vi "controllerFPGA_multiTarget.vi"() -> ()   [LabVIEW 2016]
uses:
  <vilib>/Platform/TimedLoop/XDataNode/timing_clust.ctl
  <vilib>/Platform/TimedLoop/XDataNode/nitl_modes.ctl
  <vilib>/Platform/TimedLoop/XDataNode/wakeup.ctl
  <vilib>/rvi/Emulation/niFpgaGetClockAttributes.vi
  <vilib>/rvi/Emulation/niFpgaSctlEmulationGetInTimedLoop.vi
  <vilib>/rvi/Emulation/niFpgaEmulationReportErrorSimple.vi
  <vilib>/rvi/Memory/Memory_Emulation/nirvimemoryFastEmulation.vi
  <vilib>/rvi/Memory/Memory_Emulation/nirvimemoryEmulation.vi
  <vilib>/rvi/Emulation/niFpgaEmulationIsFPGAContextNoSignature.vi
  <vilib>/rvi/DataTransferAndStorage/Container/Common/niFpgaContainerGetUniqueNameForEmu.vi
  <vilib>/rvi/Emulation/niFpgaProcessEmulError.vi
  <vilib>/rvi/errors/nirviReportUnexpectedCaseInternalError (U32).vi
  <vilib>/rvi/Emulation/niFpgaCriticalErrorInLSC.vi
  <vilib>/rvi/errors/niFpgaSetErrorForExecOnDevCompSimple.vi
  <vilib>/rvi/eio/common/nirviEmuReportErrorAndStop.vi
  <vilib>/rvi/FIFO/Fifo_Resource/nirvififoEmulationSetSize.vi
  <vilib>/rvi/FIFO/Fifo_Resource/nirviFifoEmulationQueueMgr.vi
  <instcachedir>/0/nirviFifoEmulationQueueMgr_E5CAEC123FF24DC58D834DCA3CDAA9B5.lvgen/nirviFifoEmulationQueueMgr_E5CAEC123FF24DC58D834DCA3CDAA9B5_010.vi
  <vilib>/Utility/error.llb/Clear Errors.vi
  <vilib>/rvi/FIFO/Fifo_Resource/nirvififoEmulationCreateLock.vi
  <vilib>/rvi/FIFO/Fifo_Resource/nirvififoEmulationObtainLock.vi
  <vilib>/rvi/FIFO/Fifo_Resource/nirvififoEmulationReleaseLock.vi
  <vilib>/rvi/occurrence/nirviWaitOnOccurrenceBase.vi
  <vilib>/rvi/errors/nirviReportUnexpectedCaseInternalError.vi
  <vilib>/rvi/FIFO/Fifo_Resource/nirvififoEmulationDetermineInputValidOut.vi
  <vilib>/rvi/Memory/Memory_Emulation/niFpgaMemoryEmulationCacheClearOnFirstRun.vi
  <vilib>/rvi/Memory/Memory_Emulation/nirvimemoryEmulationManagerCache_MakeExclusive.vi
  <vilib>/rvi/Memory/Memory_Emulation/niFpgaMemoryEmulationValidateCache.vi
  <vilib>/rvi/Memory/Memory_Emulation/nirvimemoryEmulationManagerCache_InsertValue.vi
  <vilib>/rvi/Memory/Memory_Emulation/nirvimemoryEmulationManagerCache_ReleaseExclusive.vi
  <vilib>/rvi/Memory/Memory_Emulation/nirvimemoryEmulationManagerCache_GetValue.vi
  <vilib>/rvi/Memory/Memory_Emulation/nirvimemoryEmulationManagerCache_SetValue.vi
  <vilib>/rvi/eio/common/nirviEmuTemplateMethod_errors.vi
  <instcachedir>/0/nirviFifoEmulationQueueMgr_E5CAEC123FF24DC58D834DCA3CDAA9B5.lvgen/nirviFifoEmulationQueueMgr_E5CAEC123FF24DC58D834DCA3CDAA9B5_009.vi
  <instcachedir>/0/nirviFifoEmulationQueueMgr_E5CAEC123FF24DC58D834DCA3CDAA9B5.lvgen/nirviFifoEmulationQueueMgr_E5CAEC123FF24DC58D834DCA3CDAA9B5_021.vi
  <instcachedir>/0/nirviFifoEmulationQueueMgr_E5CAEC123FF24DC58D834DCA3CDAA9B5.lvgen/nirviFifoEmulationQueueMgr_E5CAEC123FF24DC58D834DCA3CDAA9B5_014.vi
  <vilib>/rvi/interface/RandomDataEmulation/niFpgaRandomDataHandleErrors.vi
  <instcachedir>/0/nirviFifoEmulationQueueMgr_E5CAEC123FF24DC58D834DCA3CDAA9B5.lvgen/nirviFifoEmulationQueueMgr_E5CAEC123FF24DC58D834DCA3CDAA9B5_036.vi
  <instcachedir>/0/nirviFifoEmulationQueueMgr_E5CAEC123FF24DC58D834DCA3CDAA9B5.lvgen/nirviFifoEmulationQueueMgr_E5CAEC123FF24DC58D834DCA3CDAA9B5_035.vi
  <vilib>/rvi/eio/common/nirviEmuTemplatePropertySet_noerrors.vi
  <instcachedir>/0/nirviFifoEmulationQueueMgr_E5CAEC123FF24DC58D834DCA3CDAA9B5.lvgen/nirviFifoEmulationQueueMgr_E5CAEC123FF24DC58D834DCA3CDAA9B5_003.vi
  <instcachedir>/0/nirviFifoEmulationQueueMgr_E5CAEC123FF24DC58D834DCA3CDAA9B5.lvgen/nirviFifoEmulationQueueMgr_E5CAEC123FF24DC58D834DCA3CDAA9B5_000.vi
  <instcachedir>/0/nirviFifoEmulationQueueMgr_E5CAEC123FF24DC58D834DCA3CDAA9B5.lvgen/nirviFifoEmulationQueueMgr_E5CAEC123FF24DC58D834DCA3CDAA9B5_032.vi
  <instcachedir>/0/nirviFifoEmulationQueueMgr_E5CAEC123FF24DC58D834DCA3CDAA9B5.lvgen/nirviFifoEmulationQueueMgr_E5CAEC123FF24DC58D834DCA3CDAA9B5_007.vi
  <instcachedir>/0/nirviFifoEmulationQueueMgr_E5CAEC123FF24DC58D834DCA3CDAA9B5.lvgen/nirviFifoEmulationQueueMgr_E5CAEC123FF24DC58D834DCA3CDAA9B5_011.vi
  <instcachedir>/0/nirviFifoEmulationQueueMgr_E5CAEC123FF24DC58D834DCA3CDAA9B5.lvgen/nirviFifoEmulationQueueMgr_E5CAEC123FF24DC58D834DCA3CDAA9B5_004.vi
  <instcachedir>/0/nirviFifoEmulationQueueMgr_E5CAEC123FF24DC58D834DCA3CDAA9B5.lvgen/nirviFifoEmulationQueueMgr_E5CAEC123FF24DC58D834DCA3CDAA9B5_033.vi
  <vilib>/rvi/DataTransferAndStorage/Container/XNode/niFpgaContainer.xnode
  <vilib>/Platform/TimedLoop/XDataNode/XDataNode.xnode
  <vilib>/rvi/FIFO/Fifo_Resource/nirvififoEmulationRead.vi
  <vilib>/rvi/FXPMathLib/FxpInterpret/XNode/nifxpmath_Interpret.xnode
  <vilib>/rvi/FIFO/Fifo_Resource/nirvififoEmulationWrite.vi
  <vilib>/rvi/DataTransferAndStorage/Register/Emulation/niFpgaRegisterEmulation.vi
  <vilib>/eio/EIONode/EIONode.xnode
  <vilib>/rvi/interface/RandomDataEmulation/nirviRandomDataFpgaReadWriteTemplate.vi
  <vilib>/eio/EIOPropertyNode/EIOPropertyNode.xnode
  <vilib>/rvi/DataTransferAndStorage/Handshake/Emulation/niFpgaHandshakeEmulation.vi
  <vilib>/rvi/FXPMathLib/FxpAdd/XNode/nifxpmath_Add.xnode
  <vilib>/Platform/TimedLoop/XDataNode/XDNodeRunTimeDep.lvlib
  <instrlib>/_niInstr/Basic Elements/v1/FPGA/niInstr Basic Elements v1 FPGA.lvlib
  <vilib>/rvi/FXPMathLib/sim/FxpSim.dll
  <vilib>/rvi/eio/common/nirviEmuTemplatePropertyGet_errors.vi
  <vilib>/rvi/eio/common/nirviEmuTemplatePropertyGet_noerrors.vi
  <vilib>/rvi/eio/common/nirviEmuTemplatePropertySet_errors.vi
  <vilib>/rvi/Memory/Memory_Emulation/niFpgaMemoryEmulationDramRetrieveData.vi
  <vilib>/rvi/Memory/Memory_Emulation/niFpgaMemoryFastEmulationDramWriteAndRequestData.vi
  <vilib>/rvi/Memory/Memory_Emulation/niFpgaMemoryEmulationDramWriteAndRequestData.vi
panel:
  in  "dio.i.dataIn":bool
  in  "dio.p.multiplexerOE":bool
  in  "dio.p.multiplexerclock":bool
  in  "dio.p.multiplexerSync":bool
  in  "dio.p.multiplexerReset":bool
  in  "se.tabs":T1(tab)
  in  "se.p.closedLoop":bool
  in  "se.p.scanSize":T2
  in  "se.p.transformMatrix":T3
  in  "se.p.scanOffsets":cluster{"x":fxp<+/-,16,1>, "y":fxp<+/-,16,1>}
  in  "se.p.clocks":T4={"outputRate"=50, "fastDecFactor"=0, "outWaveSizeFast"=0, "pplUpsampling"=0, "numLines"=0, "se.p.fastInvDec"=0.0, "se.p.slowUpStep"=0.0, "se.p.outWaveSizeSlow"=0, "blankingMax"=10000000, "se.p.fastBlanking"={"startFwd"=0, "endFwd"=10000, "startBwd"=0, "endBwd"=0, "disableBlanking"=FALSE, "useCoarseCounter"=TRUE}}
  in  "se.p.modes":T5
  in  "se.m.slowAxis":T6
  in  "se.m.fastAxis":T6
  out "se.s.realXYOutputRate":u32
  out "se.s.blankingOff":bool
  out "se.o.position":T7
  out "clocksOut":T8
  in  "se.p.durationTrigger":u16=100
  in  "se.p.y.fbParams":T9={"enable"=FALSE, "setPoint"=0.001007080078125, "pGain"=0.0, "iGain"=0.10000038146972656, "gainScale"=0}
  in  "se.p.x.fbParams":T9={"enable"=FALSE, "setPoint"=0.001007080078125, "pGain"=0.0, "iGain"=0.10000038146972656, "gainScale"=0}
  in  "se.mot.p.target":cluster{"x":fxp<+/-,16,1>, "y":fxp<+/-,16,1>}
  out "se.mot.s.running":bool
  in  "se.mot.p.clocks":T10
  in  "se.mot.m.motion":T11
  out "se.mot.s.origin":T12
  in  "se.sid.prbs":cluster{"write":bool, "index":u16, "data":bool}
  in  "se.sid.start":bool
  in  "se.sid.p.axisXNotY":bool=TRUE
  in  "se.sid.p.params":T13={"sysIdOutputRate"=100, "sysIdWaveSize"=4092, "sysIdRepetitions"=50, "high"=0.0, "low"=0.0} {"sysIdOutputRate" min=10}
  out "se.sid.s.repetitions":u16
  out "se.sid.s.running":bool
  in  "stepmot.delay(ms)":u16
  in  "stepmot.dir":bool
  in  "stepmot.enable":bool
  in  "stepmot.on":bool
  in  "stepmot.steps":u16
  in  "smd.address":i8
  in  "smd.p.writeMem":T14={"write"=FALSE, "index"=0, "data"=[TRUE, FALSE, FALSE, FALSE]}
  out "stepmot.running":bool
  in  "ort.bgc.requestType":i16(ring) items=["Never", "EndOfLine", "EndOfFrame"]
  in  "aio.wfm.enable":bool
  out "aio.s.slowActualOutputRate":u32
  in  "wfm.rampRange":T15
  in  "wfm.Parameters":T16
  in  "wfm.initialPositions":T17
  in  "wfm.reset":cluster{"rampx":bool, "ustepx":bool}
  out "wfm.displacementFinished":bool
  out "wfm.microStepIndex":cluster{"CurrentUstep":i16, "NextUstep":i16}
  out "wfm.rampIndex":cluster{"ramp index":i16, "NextRamp":i16}
  in  "Tab Control":T18(tab)
  in  "aio.o.fastInput":bool
  in  "aio.o.invertHeight":bool
  out "aio.o.inputs":i16[](array[numeric])
  out "aio.s.HSaux":fxp<+/-,24,16>
  in  "aio.i.slowInputRate":u16 caption="Count(Ticks)"
  out "aio.s.slowVertical":i16
  out "aio.s.sum":i16
  out "aio.s.slowHoriz":i16
  in  "aio.o.bypassDither":bool
  in  "aio.m.drive":cluster{"write":bool, "data":i16, "index":u16}
  in  "aio.o.disableExc":bool=TRUE
  out "aio.s.clock":refnum<k21>
  out "aio.s.slowActualInputRate":u32
  out "aio.s.slowActualFBOutRate":u32
  in  "aio.o.invertOutputs":bool[](array[boolean])=[FALSE, FALSE, FALSE, FALSE, FALSE, FALSE, FALSE, FALSE]
  in  "aio.o.outputs":i16[](array[numeric])=[0, 0, 0, 0]
  in  "aio.o.invertInputs":bool[](array[boolean])=[FALSE, FALSE, FALSE, FALSE, FALSE, FALSE, FALSE, FALSE]
  in  "aio.o.invert2Inputs":bool[](array[boolean])=[FALSE, FALSE]
  in  "aio.i.samplingDecimation":u16=1
  in  "AI.voltage Range":T19(ring)
  in  "aio.p.fastADCclockdec":u16
  out "aio.s.fastVertical":i16
  out "aio.s.fastHoriz":i16
  in  "aio.o.heightLimits":cluster{"upper":i16, "lower":i16}={"upper"=32767, "lower"=-32768}
  in  "aio.flt.bypass":bool[](array[boolean])=[TRUE, TRUE, TRUE, TRUE]
  in  "aio.flt.p.anot4x":fxp<+/-,24,8>[](array[numeric])=[0.0, 0.0, 0.0, 0.0, 0.0, 0.0, 0.0, 0.0]
  in  "aio.flt.p.b4x":fxp<+/-,24,8>[](array[numeric])=[0.0, 0.0, 0.0, 0.0, 0.0, 0.0, 0.0, 0.0, 0.0, 0.0, 0.0, 0.0]
  in  "hdt.aux.o.enable":bool
  in  "hdt.o.enable":bool=TRUE
  out "hdt.o.overflow":bool
  out "hdt.o.ticksPerPixel":u32
  in  "hdt.mainOutStreamSelect":u8(ring) items=["PID/ORT", "SICM"]
  out "hdt.int.s.debug":T20
  in  "hdt.int.p.memWriteSource":u8(ring) items=["ORT", "SICM"]
  out "hdt.int.s.dataLost":bool
  in  "hdt.int.s.clearDataLost":bool
  in  "hdt.int.p.readParams":T21={"hdt.int.s.transferSource"=0, "hdt.int.p.useInternalMemStartPos"=FALSE, "hdt.int.p.memStartPos"=0.0, "hdt.int.p.readLength"=100, "hdt.int.p.readFwd"=TRUE, "hdt.int.p.memReadDec"=10, "hdt.int.p.startTransfer"=TRUE} {"hdt.int.s.transferSource" items=["memoryChan1", "memoryChan2", "processVarFixedNoPts", "processVarStream", "systemId", "interleaveMemCh1Ch2"]}
  out "hdt.debugStream":T22
  in  "hdt.p.mainAverageEnabled":bool=TRUE
  in  "fb.p.limits":T23={"upperLimit"=1.0, "lowerLimit"=-1.0}
  in  "fb.i.source":u8(ring) items=["Contact Mode", "ORT", "Aux"]
  in  "fb.p.enable":bool
  in  "fb.p.params":T24={"setPoint"=0.001007080078125, "pGain"=0.0, "iGain"=0.10000038146972656, "gainScale"=3, "setPointAlt"=0.001007080078125}
  in  "fb.loff.p.params":T25={"liftHeight"=0.0498046875, "disengagePos"=-1.0}
  out "fb.s.atLimit":bool
  out "fb.i.rescaled":fxp<+/-,24,1> format="%#_6p"
  out "fb.i.raw":fxp<+/-,24,16>
  in  "fb.p.allowSetpointSwitch":bool
  out "fb.mot.s.running":bool
  out "fb.o.height":fxp<+/-,31,4>
  in  "fb.mot.m.motion":T26
  in  "fb.zWatchdogArm":bool=TRUE
  in  "fb.p.zWatchDogTreshold":fxp<+/-,20,2>
  in  "fb.mot.p.params":T27
  in  "ort.p.waveSize":u16=5000
  in  "ort.o.piezoMode":bool
  in  "ort.p.methodParams":T28={"ort.p.winSizeP2"=2, "ort.p.syncPoint"=0, "ort.p.useSyncPoint"=FALSE, "ort.p.bypassAvg"=FALSE, "ort.p.searchBounds"={"maxSearchLower"=200, "maxSearchUpper"=600}}
  out "ort.o.maxIndex":u16
  in  "ort.p.fcAvgEnable":bool
  in  "ort.p.fcAvg":i8=-4
  in  "ort.bgc.p.scannerTc":u32=1000 caption="scanner Time Constant [us]"
  in  "ort.bgc.p.start":bool
  in  "ort.bgc.p.bgCntP2":u16=12
  in  "ort.bgc.p.waitTicks":u32
  in  "itc.p.allowBGC":bool
  out "aio.s.ortSubstDeflection":cluster{"index":u16, "data":i16}
  out "ort.o.interactionMax":fxp<+/-,24,16>
  in  "ort.fit.p.params":T29={"maxLoc"=0, "threshold"=0, "fitHardPtLimit"=5000}
  in  "ort.fit.m.coefficients":T30
  in  "ort.fit.m.weights":T31
  in  "hsdc.p.points":u32
  in  "hsdc.p.start":bool
  in  "hsdc.o.address":u32
  out "hsdc.o.read":T32
  in  "hsdc.p.substBgnd":bool=TRUE
  in  "sid.m.motion":cluster{"write":bool, "data":bool, "index":u16}
  out "sid.s.running":bool
  out "sid.o.count":u16
  in  "sid.p.start":bool
  in  "sid.p.params":T33={"sysIdOutputRate"=100, "sysIdWaveSize"=4092, "sysIdRepetitions"=50, "lowValue"=0.0, "highValue"=0.010009765625} {"sysIdOutputRate" min=10}
  in  "sid.allowExternalRecord":bool=TRUE
  in  "sid.p.idSource":u8(ring) items=["error", "height"]
  in  "sicm.m.upMotion":T26
  out "sicm.o.height":fxp<+/-,28,2>
  in  "sicm.blc.p.params":T34={"se.blc.p.postRetractDelay"=0, "se.blc.p.windowSize"=0, "se.blc.p.updateFactor"=-8, "blc.resetBackground"=FALSE, "se.blc.p.mindelta"=3.0502676963806152e-05}
  in  "sicm.p.clocks":T35
  in  "sicm.p.params":T36={"sicm.p.setPoint"=0.9999847412109375, "sicm.p.setPointFrac"=1.0, "stepDown"=0.0, "retractHeight"=0.0, "adaptiveMin"=0.0} {"sicm.p.setPoint" format="%#_3g"}
  in  "sicm.display":T37
  in  "sicm.p.modes":T38
  out "sicm.Debug":T39
  out "sicm.s.baseline":T40
  out "sicm-hdt.t.triggerHeight":fxp<+/-,22,4>
  out "flt.o.height":fxp<+/-,20,2>
  in  "flt.ss.p.enable":bool
  in  "flt.ss.p.rate":u16=1000
  in  "flt.bypass1":bool[](array[boolean])=[TRUE, TRUE, TRUE, TRUE, TRUE, TRUE, TRUE, TRUE]
  in  "flt.bypass2":bool[](array[boolean])=[TRUE, TRUE, TRUE, TRUE]
  in  "flt.p.anot8x":fxp<+/-,24,8>[](array[numeric])=[0.0, 0.0, 0.0, 0.0, 0.0, 0.0, 0.0, 0.0, 0.0, 0.0, 0.0, 0.0, 0.0, 0.0, 0.0, 0.0]
  in  "flt.p.b8x":fxp<+/-,24,8>[](array[numeric])=[0.0, 0.0, 0.0, 0.0, 0.0, 0.0, 0.0, 0.0, 0.0, 0.0, 0.0, 0.0, 0.0, 0.0, 0.0, 0.0, 0.0, 0.0, 0.0, 0.0, 0.0, 0.0, 0.0, 0.0]
  in  "flt.p.anot4x":fxp<+/-,24,8>[](array[numeric])=[0.0, 0.0, 0.0, 0.0, 0.0, 0.0, 0.0, 0.0]
  in  "flt.p.b4x":fxp<+/-,24,8>[](array[numeric])=[0.0, 0.0, 0.0, 0.0, 0.0, 0.0, 0.0, 0.0, 0.0, 0.0, 0.0, 0.0]
  in  "flt.bypassPI":bool
  in  "flt.i.bypassSource":u8(ring) items=["process Variable", "SICM", "ramp"]
  in  "flt.o.hold":bool
  out "rmp.s.running":bool
  in  "rmp.p.params":T41={"rmp.p.downRate"=0.0, "rmp.p.upRate"=0.0, "rmp.p.startPos"=0.0, "rmp.p.clockDec"=40, "rmp.p.recordClockDec"=100, "rmp.p.enableHDTPointRecord"=FALSE, "rmp.p.pull"=FALSE}
  in  "rmp.p.triggerParams":T42={"rmp.triggerSource"=0, "rmp.p.triggerPositive"=TRUE, "rmp.p.triggerLevel"=0.0} {"rmp.triggerSource" items=["Absolute z height", "Process variable", "External"]}
  in  "rmp.p.useIntHeightAsStart":bool
  in  "rmp.p.action":cluster{"rmp.p.start":bool, "rmp.p.stop":bool}
  in  "rmp.p.reset":T43
  in  "lwr.p.avgCnt":u8
  in  "lwr.p.readAddress":u16
  out "lwr.o.readData":i32
  in  "lwr.p.start":bool
  # "Scan Engine"
  # "Manual positioning of the tip in XY direction"
  # "Stepper motor driver"
  # "Stepper Motor Driver\ninterface"
  # "inter target communication"
  # "Analog I/O"
  # "Data transfer to host"
  # "Feedback (PI)"
  # "Off-resonance tapping"
  # "ort.bgc: Background correction for ORT"
  # "Curve fitting parameters for ORT material property measurement"
  # "High-speed data capture"
  # "System Identification"
  # "Requirements for SICM: flt.bypassPI = TRUE || hdt.mainOutStreamSelect = SICM || sicm.p.setPointFrac = 1/(setpoint-1)"
  # "Filtering of in- and outputs"
  # "Local wave recording"
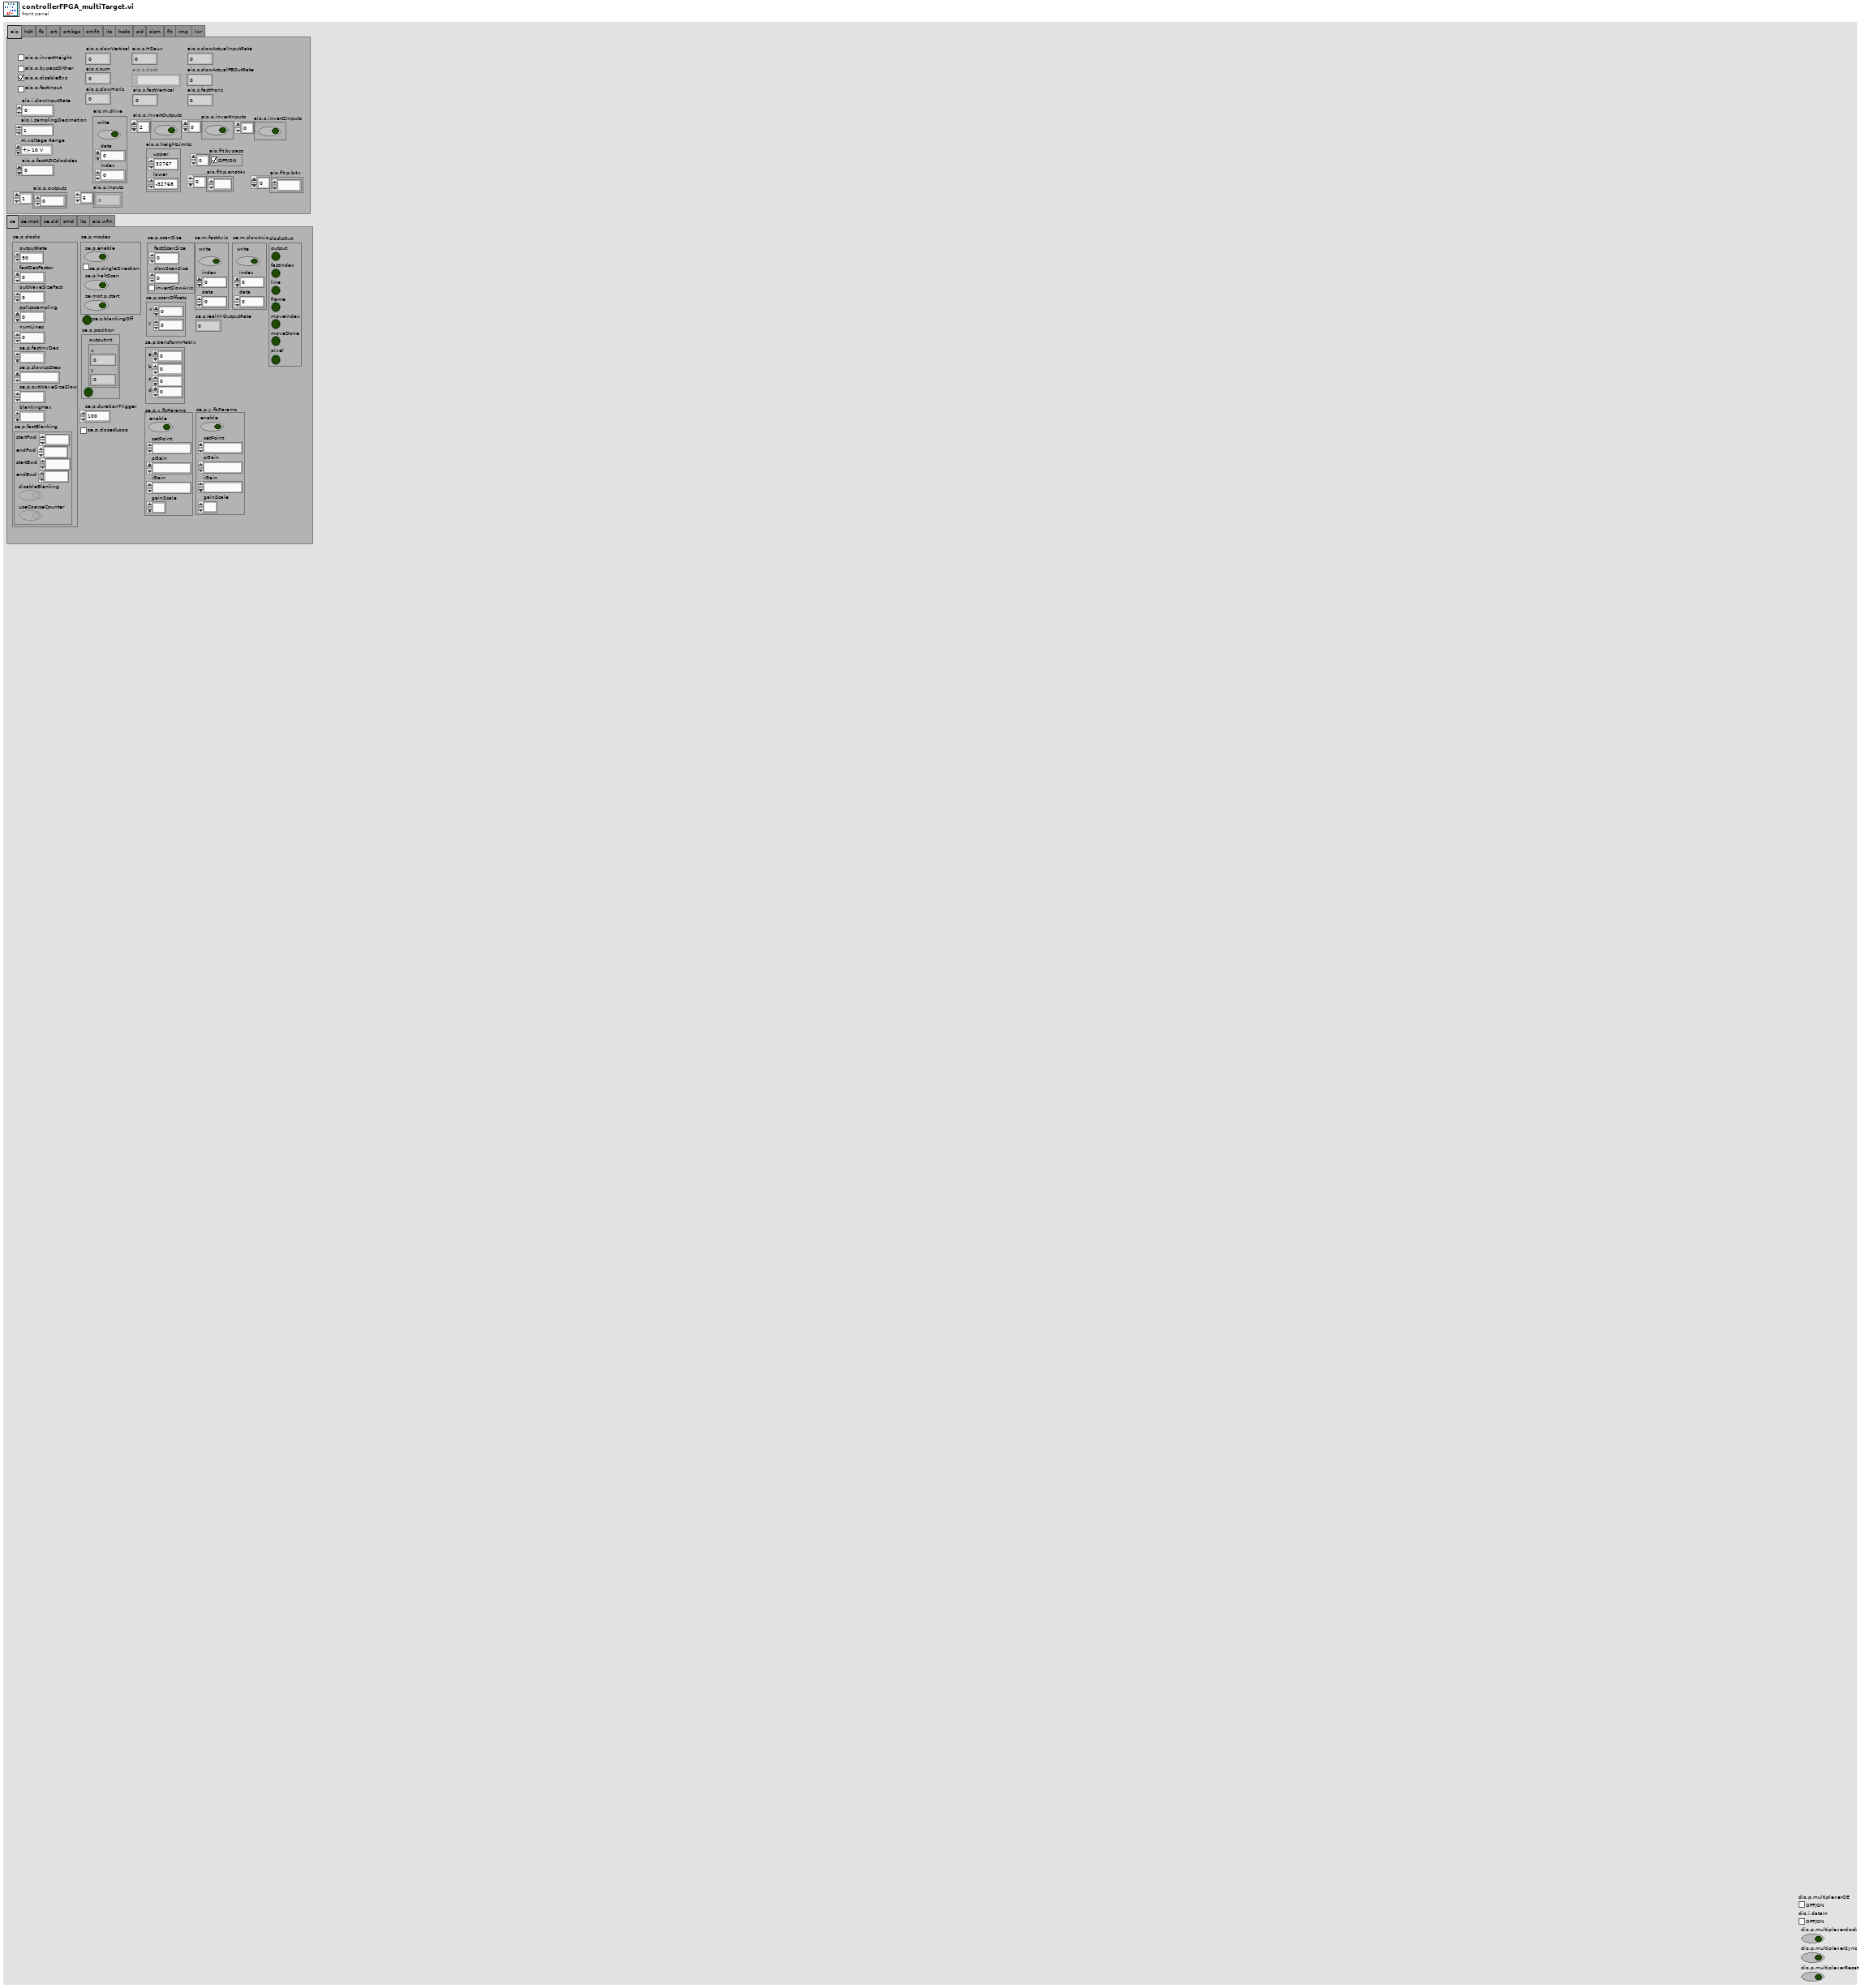
[diagram p1: front panel]
types:
  T1 = enum32{"se", "se.mot", "se.sid", "smd", "itc", "aio.wfm"}
  T2 = cluster{"fastScanSize":fxp<+,17,1>, "slowScanSize":fxp<+,17,1>, "invertSlowAxis":bool}
  T3 = cluster{"a":fxp<+/-,18,2>, "b":fxp<+/-,18,2>, "c":fxp<+/-,18,2>, "d":fxp<+/-,18,2>}
  T4 = cluster{"outputRate":u16, "fastDecFactor":u16, "outWaveSizeFast":u16, "pplUpsampling":u16, "numLines":u16, "se.p.fastInvDec":fxp<+,22,0>, "se.p.slowUpStep":fxp<+,28,0>, "se.p.outWaveSizeSlow":u16, "blankingMax":u32, "se.p.fastBlanking":cluster{"startFwd":u32, "endFwd":u32, "startBwd":u32, "endBwd":u32, "disableBlanking":bool, "useCoarseCounter":bool}}
  T5 = cluster{"se.p.enable":bool, "se.p.singleDirection":bool, "se.p.haltScan":bool, "se.mot.p.start":bool}
  T6 = cluster{"write":bool, "index":u16, "data":fxp<+/-,18,2>}
  T7 = cluster{"outputInt":cluster{"x":i16, "y":i16}, bool}
  T8 = cluster{"output":bool, "fastIndex":bool, "line":bool, "frame":bool, "moveIndex":bool, "moveDone":bool, "pixel":bool}
  T9 = cluster{"enable":bool, "setPoint":fxp<+/-,17,1>, "pGain":fxp<+/-,20,4>, "iGain":fxp<+/-,20,1>, "gainScale":i8}
  T10 = cluster{"moveToDecFactor":u16, "moveToWaveSize":u16, "se.mot.p.invDec":fxp<+,16,0>}
  T11 = cluster{"write":bool, "index":u16, "data":fxp<+/-,18,1>}
  T12 = cluster{"xOut":fxp<+/-,18,2>, "yOut":fxp<+/-,18,2>}
  T13 = cluster{"sysIdOutputRate":u16, "sysIdWaveSize":u16, "sysIdRepetitions":u16, "high":fxp<+/-,17,1>, "low":fxp<+/-,17,1>}
  T14 = cluster{"write":bool, "index":u16, "data":bool[]}
  T15 = cluster{"min_x":i16, "max_x":i16, "Total number of ramps":i16, "OutputScale":fxp<+/-,16,16>, "Steps in a ramp":i16}
  T16 = cluster{"target ":i16, "increment":i16, "ClockDivider":i16, "axis":enum16{"none", "x", "y", "z"}}
  T17 = cluster{"InitialX":fxp<+/-,16,16>, "InitialY":fxp<+/-,16,16>, "InitialZ":fxp<+/-,16,16>}
  T18 = enum32{"aio", "hdt", "fb", "ort", "ort.bgc", "ort.fit", "itc", "hsdc", "sid", "sicm", "flt", "rmp", "lwr"}
  T19 = enum8{"+/- 10 V", "+/- 5 V", "+/- 2 V", "+/- 1 V"}
  T20 = cluster{"Data":u16, cluster{"Element":i16, "Output Valid":bool}}
  T21 = cluster{"hdt.int.s.transferSource":u8, "hdt.int.p.useInternalMemStartPos":bool, "hdt.int.p.memStartPos":fxp<+,14,14>, "hdt.int.p.readLength":u16, "hdt.int.p.readFwd":bool, "hdt.int.p.memReadDec":u16, "hdt.int.p.startTransfer":bool}
  T22 = cluster{"ch2":fxp<+/-,22,1>, "ch3":fxp<+/-,22,1>}
  T23 = cluster{"upperLimit":fxp<+/-,28,4>, "lowerLimit":fxp<+/-,28,4>}
  T24 = cluster{"setPoint":fxp<+/-,17,1>, "pGain":fxp<+/-,20,4>, "iGain":fxp<+/-,20,1>, "gainScale":i8, "setPointAlt":fxp<+/-,17,1>}
  T25 = cluster{"liftHeight":fxp<+/-,15,4>, "disengagePos":fxp<+/-,22,1>}
  T26 = cluster{"write":bool, "data":fxp<+,16,1>, "index":u16}
  T27 = cluster{"enableManualMotion":bool, "doMove":bool, "integratorTarget":fxp<+/-,22,2>, "clocks":cluster{"inverseDecimation":fxp<+,22,0>, "decimation":u16, "waveSize":u16, "pixelDecimation":u16}}
  T28 = cluster{"ort.p.winSizeP2":u16, "ort.p.syncPoint":u16, "ort.p.useSyncPoint":bool, "ort.p.bypassAvg":bool, "ort.p.searchBounds":cluster{"maxSearchLower":u16, "maxSearchUpper":u16}}
  T29 = cluster{"maxLoc":u16, "threshold":i16, "fitHardPtLimit":u16}
  T30 = cluster{"write":bool, "index":u16, "fitCoefficients":cluster{"a":fxp<+/-,21,7>, "b":fxp<+/-,21,7>, "factorA":i8, "factorB":i8}}
  T31 = cluster{"write":bool, "data":fxp<+,20,0>, "index":u16}
  T32 = cluster{"Element 1":i16, "Element 2":i16, "Element 3":i16, "Element 4":i16}
  T33 = cluster{"sysIdOutputRate":u16, "sysIdWaveSize":u16, "sysIdRepetitions":u16, "lowValue":fxp<+/-,16,1>, "highValue":fxp<+/-,16,1>}
  T34 = cluster{"se.blc.p.postRetractDelay":u16, "se.blc.p.windowSize":u16, "se.blc.p.updateFactor":i16, "blc.resetBackground":bool, "se.blc.p.mindelta":fxp<+/-,12,-14>}
  T35 = cluster{"inverseDecimation":fxp<+,22,0>, "decimation":u16, "waveSize":u16, "pixelDecimation":u16}
  T36 = cluster{"sicm.p.setPoint":fxp<+,20,0>, "sicm.p.setPointFrac":fxp<+/-,20,14>, "stepDown":fxp<+/-,28,4>, "retractHeight":fxp<+/-,28,4>, "adaptiveMin":fxp<+,10,0>}
  T37 = cluster{"sicm.ptsAfterTrig":u16, "sicm.p.memorywWriteDec":u16}
  T38 = cluster{"sicm.p.enable":bool, "sicm.p.adaptiveStepDown":bool, "sicm.p.relSetpoint":bool}
  T39 = cluster{"retractHeight":fxp<+/-,31,4>, "interpOutput":fxp<+/-,19,2>, "x+y":fxp<+/-,28,1>}
  T40 = cluster{"carryOut":fxp<+/-,22,2>, "1/x":fxp<+/-,32,24>, "x*y":fxp<+,24,1>}
  T41 = cluster{"rmp.p.downRate":fxp<+/-,22,-10>, "rmp.p.upRate":fxp<+/-,22,-10>, "rmp.p.startPos":fxp<+/-,24,2>, "rmp.p.clockDec":u16, "rmp.p.recordClockDec":u16, "rmp.p.enableHDTPointRecord":bool, "rmp.p.pull":bool}
  T42 = cluster{"rmp.triggerSource":u8, "rmp.p.triggerPositive":bool, "rmp.p.triggerLevel":fxp<+/-,24,16>}
  T43 = cluster{"rmp.p.resetStartPos":bool, "rmp.p.resetEndPos":bool}
  T44 = typedef "XDNodeRunTimeDep.lvlib/timing_clust.ctl" = cluster{"Expected End [f-1]":u64, "Actual End [f-1]":u64, "Finished Late? [f-1]":bool, "Expected End [i-1]":u64, "Actual End [i-1]":u64, "Finished Late? [i-1]":bool, "Expected Start [i]":u64, "Actual Start [i]":u64, "Expected Start [f]":u64, "Actual Start [f]":u64, "Source Name":string, "Structure Name":string, "Period":i64, "Deadline":i64, "Offset":i64, "Start":i64, "Priority":i32, "Timeout":i32, "Mode":T45, "Wakeup Reason":T46, "Error":errorcluster, "Source Type":string, "Secondary Source Type":string, "Global End Time":u64, "Global Start Time":u64, "Frame Duration":u64, "Iteration Duration":u64, "Assigned CPU":i32, "I/O Scan Engine Mode":u32}
  T45 = typedef "XDNodeRunTimeDep.lvlib/nitl_modes.ctl" = enum32{"No Change", "Process missed periods, maintain original phase", "Discard missed periods, maintain original phase", "Process missed periods, ignore original phase", "Discard missed periods, ignore original phase"}
  T46 = typedef "XDNodeRunTimeDep.lvlib/wakeup.ctl" = enum32{"Normal", "Aborted", "Asynchronous wakeup", "Timing source error", "Timed loop error", "Timeout"}
  T47 = cluster{"se.p.scanOffsets":cluster{"x":fxp<+/-,16,1>, "y":fxp<+/-,16,1>}, "se.p.transformMatrix":cluster{"a":fxp<+/-,18,2>, "b":fxp<+/-,18,2>, "c":fxp<+/-,18,2>, "d":fxp<+/-,18,2>}, "se.p.scanSize":cluster{"fastScanSize":fxp<+,17,1>, "slowScanSize":fxp<+,17,1>, "invertSlowAxis":bool}}
  T48 = cluster{"se.mot.p.clocks":cluster{"moveToDecFactor":u16, "moveToWaveSize":u16, "se.mot.p.invDec":fxp<+,16,0>}, "se.p.clocks":cluster{"outputRate":u16, "fastDecFactor":u16, "outWaveSizeFast":u16, "pplUpsampling":u16, "numLines":u16, "se.p.fastInvDec":fxp<+,22,0>, "se.p.slowUpStep":fxp<+,28,0>, "se.p.outWaveSizeSlow":u16, "blankingMax":u32, "se.p.fastBlanking":cluster{"startFwd":u32, "endFwd":u32, "startBwd":u32, "endBwd":u32, "disableBlanking":bool, "useCoarseCounter":bool}}}
  T49 = cluster{"outputInt":cluster{"y":fxp<+/-,16,1>, "y":fxp<+/-,16,1>}, bool}
  T50 = cluster{"x+y":fxp<+/-,18,2>, "x+y":fxp<+/-,18,2>}
  T51 = cluster{"outputInt":cluster{"sid.o.height":fxp<+/-,28,1>, "sid.o.height":fxp<+/-,28,1>}, bool}
  T52 = cluster{"sid.o.height":fxp<+/-,28,1>, "sid.o.height":fxp<+/-,28,1>}
  T53 = cluster{"X":fxp<+/-,28,1>, "integer_X":i16, "error":fxp<+/-,25,2>}
  T54 = cluster{"liftHeight":fxp<+/-,15,4>, "disengagePos":fxp<+/-,22,1>, "liftOff":bool}
  T55 = cluster{"Element":fxp<+/-,22,4>, "Output Valid":bool}
  T56 = cluster{"Element":fxp<+/-,24,16>, "Output Valid":bool}
  T57 = cluster{"stepDown":fxp<+/-,28,4>, "x+y":fxp<+/-,20,1>, "x+y":fxp<+/-,28,1>}
  T58 = cluster{"x-y":fxp<+/-,22,4>, "output valid":bool}
  T59 = cluster{"x+y":fxp<+/-,28,2>, "output valid":bool}
  T60 = cluster{"zHeight":fxp<+/-,28,1>, "integer_zHeight":i16, "error":fxp<+/-,25,2>, "pidAtLimit":bool, "moving":bool}
  T61 = cluster{"rmp.o.height":fxp<+/-,24,2>, "rmp.o.valid":bool}
  T62 = cluster{"Element":fxp<+/-,27,4>, "rmp.o.valid":bool}[]
  T63 = cluster{"Element":fxp<+/-,27,4>, "rmp.o.valid":bool}
  T64 = cluster{"error":fxp<+/-,25,2>, "output valid":bool}
  T65 = cluster{"zHeight":fxp<+/-,31,4>, "output valid":bool}
  T66 = cluster{"zHeight":fxp<+/-,31,4>, "output valid":bool}[]
  T67 = cluster{"index":u16, "data":i16, "background":i16, "outptValid":bool}
  T68 = cluster{"cycleMax":fxp<+/-,24,16>, "outputValid":bool}
  T69 = cluster{"index":u16, "data":i16, "background":i16, "inElementValid":bool}
  T70 = cluster{"cycleMax":fxp<+/-,24,16>, "maxPulse":bool}[]
  T71 = cluster{"cycleMax":fxp<+/-,24,16>, "maxPulse":bool}
  T72 = cluster{"index":u16, cluster{"data":i16, "background":i16}}
  T73 = cluster{"a":fxp<+/-,21,7>, "b":fxp<+/-,21,7>, "factorA":i8, "factorB":i8}
  T74 = cluster{"Xout":fxp<+/-,16,16>, "Yout":fxp<+/-,16,16>, "Zout":fxp<+/-,16,16>, "OutputValid":bool}
  T75 = cluster{"[0]":bool, "[1]":bool, "[2]":bool, "[3]":bool, "[4]":bool, "[5]":bool, "[6]":bool, "[7]":bool, "[8]":bool}
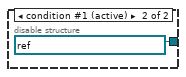
[diagram p7: hidden frame]
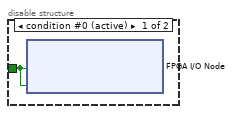
[diagram p9: hidden frame]
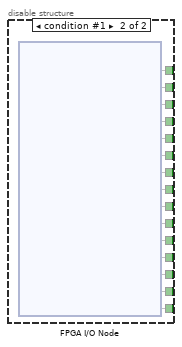
[diagram p11: hidden frame]
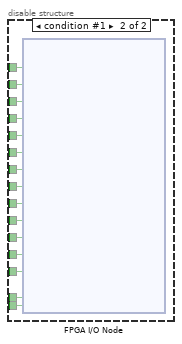
[diagram p12: hidden frame]
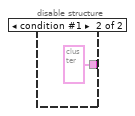
[diagram p19: hidden frame]
diagram:
  # "ts: target scope"
  # "08.09.2017"
  # "aio: Analog I/O\nName\tDescription\tLimit\naio.i.invertDeflection\tInvert the deflection input\t\naio.i.zeroDeflection\tGround the cantilever deflection input\t\naio.i.zeroAux\tGround the auxiliary controller input, usually the lateral deflection\t\naio.i.invertAux\tInvert the auxiliary input\t\naio.o.invertHeight\tInvert the height output\t\naio.o.bypassDither\tDisable the output dithering (trades speed for more resolution)\tOnly FlexRIO\naio.o.disableExc\tDisable the excitation (ORT drive or cantilever shake)\t\naio.i.slowInputRate\tSets the input sampling rate of the controller in ticks per sample, 40MHz base clock\tOnly USB-RIO\naio.o.ao4\tCheap host-controlled analog output on AO4, intended as signal or bias generator\tNot FlexRIO\naio.s.slowVertical\tVertical (normal) cantilever signal for alignment crosshair\tNot FlexRIO\naio.s.sum\tSum signal for alignment crosshair\tNot FlexRIO\naio.s.slowHoriz\tHorizontal (lateral) cantilever signal for alignment crosshair\tNot FlexRIO\naio.s.HSaux\tAuxiliary input display for sporadic display\t\naio.m.drive\tMemory access node for drive waveform\t\n\n\nhdt: Data transfer to host\nName\tDescription\tLimit\nhdt.o.overflow\tEnable the main image stream to the host\t\nhdt.aux.o.enable\tEnable the secondary image stream to the host\tNot FlexRIO\nhdt.o.overflow\tIndicates a time-out when sending image data to the host\t\nhdt.o.ticksPerPixel\tEffective, measured elapsed ticks per transferred pixel of the main image stream\nhdt.mainOutStreamSelect  PID:ORT or SICM\nhdt.int.p..readParams.\nhdt.int.s.transferSource  memoryChan1 for Interaction Curve\nmemoryChan2 for Background\nProcessVarFixNoPts: for Oscillo\nProcessVarStream: For Oscillo\nhdt.int.p.memWriteSource: ORT/SICM\n\nfb: Feedback (PI)\nName\tDescription\tLimit\nfb.p.enable\tTurn on all feedback related functions\t\nfb.p.params\tParameters for PI controller, such as setpoint, P and I gains. \ngainScale is an additional power-of-two compression factor for very large or very small gains. \nsetPointAlt is a scan-engine switchable alternative setpoint for nanomanipulation\t\nfb.loff.p.params\tRetract height for local lift-off and controller off-state output\t\nfb.i.source\tFeedback source. Effectively the mode selection for contact, ORT, AM-AFM etc.\t\nfb.s.atLimit\tIndicates a railing controller\t\nfb.i.raw\tThe current input to the PI controller, 16-bit word length\t\nfb.i.rescaled\tThe current input to the PI controller, normalized to ±1\t\nfb.o.height\tIndicates the current height of the PI controller. Used for user z position display on host\t\nfb.mot.s.running\tIndicates that a manually controlled motion in z is in progress\t\nfb.mot.p.params\tParameters for manually controlled z-motion. \nintegratorTarget is from 0 (completely retracted) to 2 (fully extended). \nmoveDecimation is the delay between points of the motion waveform, clocked the same as the PI controller.\t\nfb.mot.m.motion\tMemory acccess node for the manual z-motion\t\n\n\nort: Off-resonance tapping\nName\tDescription\tLimit\nort.p.waveSize\tSize of the excitation drive waveform. \nOn FlexRIO systems defines the tapping rate by decimating the analog I/O sampling rate.\t\nort.o.piezoMode\tEnables conventional ORT actuation by piezo \ninstead of using the drive line of the AFM for excitation (typically PORT)\t\nort.o.maxIndex\tIndex of last detected maximum force value when not using synchronous detection (useSyncPoint)\t\nort.p.methodParams\tGeneral parameters for ORT operation. \nIf synchronous detection is used, a window of 2^syncAverageBand around syncPoint is averaged and used as feedback. \nThe averaging can be disabled with the bypassAvg switch. \nIf synchronous detection is disabled, a window in ort.p.searchBounds is sequentially searched for the largest value\t\nort.p.winSizeP2\t\nort.bgc.p.readAddress\tAddress to access the internal memory for the cantilever (corrected) background motion \nand a saved interaction curve\t\nort.bgc.o.bgnd\tReturn value for reading the background at the cycle-time indicated in ort.bgc.p.readAddress\t\nort.o.interaction\tReturn value for reading the interaction at the cycle-time indicated in ort.bgc.p.readAddress\t\nort.p.fcAvgEnable\tCycle-indexed exponential moving average filter for the interaction waveform. \nUsed for display and mechanical property calculation\t\nort.p.fcAvg\tUpdate multiplier for force-time interaction curve MA filter, in power-of-two. -4 = 1/16 update\t\nort.o.sendCurve\tHost control to request a force curve to be sent over the DMA FIFO\t\nort.p.syncDecimation\tNumber of cycles between saving a force-time interaction curve to memory to be sent to the host\t\n\n\nort.bgc: Background correction for ORT\nName\tDescription\tLimit\nort.bgc.p.start\tStart the background acquisition and correction process\t\nort.bgc.p.scannerTc\tTime constant of the scanner in microseconds. \nDelay time before background motion cycles are getting accumulated for averaging.\t\nort.bgc.p.bgCntP2\tPower-of-two count of how many cycles background to acquire and average.\t\nort.bgc.p.waitTicks\tCalculated number of ticks before feedback gets re-enabled. \nThis is set as the product of ticks per output, ticks per cycle and number of background cycles that get acquired\t\nitc.p.allowBGC\tEnable or disable externally controlled requests for a correction of the background \n(usually by the scan engine at the end of a frame)\t\naio.s.ortSubstDeflection\tCurrent index and value after background correction. Typically only for debug purposes.\t\nort.o.interactionMax\tMaximum force per cycle calculated by the ORT engine for slow display or debugging, not for feedback.\t\n\n\nort.fit: Curve fitting parameters for ORT material property measurement\nName\tDescription\tLimit\nort.fit.p.params\tCurve fitting parameters. \nmaxLoc is the cycle-indexed assumed turnaround point (point of maximum force), \nthreshold is the force value used to terminate the fit \nand fitHardPtLimit is the maximum number of points that are considered before the fit is terminated, \nif not already done so by threshold.\t\nort.fit.m.coefficients\tMemory access node to write in the factors for calculating the slope from the fit accumulators\t\nort.fit.m.weights\tMemory access node for the weights of the weighted accumulator used in the slope fitting module\t\n\n\nhsdc: High-speed data capture\nName\tDescription\tLimit\nhsdc.p.points\tNumber of points to aquire\tOnly FlexRIO\nhsdc.p.start\tStarts the aquisition\tOnly FlexRIO\nhsdc.p.substBgnd\tEnable to record background corrected deflection signals. If unchecked, records raw deflection input\tOnly FlexRIO\nhsdc.o.address\tAddress to read aquired time traces from memory\tOnly FlexRIO\nhsdc.o.read\t4-value block of saved data\tOnly FlexRIO\n\n\nsid: System Identification\nName\tDescription\tLimit\nsid.m.motion\tMemory access node for system identification output waveform (usually a pseudo-random binary signal)\t\nsid.o.count\tCount of the already acquired system identification blocks (blocksize is sid.p.params->sysIdWaveSize)\t\nsid.s.running\tIndicator whether sysId is still running\t\nsid.p.params\tOperation parameters for a system identification procedure. \nOutput is decimated by sysIdOutputRate from the IO clock (FlexRIO) or the base clock (USB-RIO). \nThere will be sysIdRepetition number of blocks of sysIdWaveSize output\t\nsid.p.start\tStarts a system identification operation.\t\n\n\nflt: Filtering of in- and outputs\nName\tDescription\tLimit\nflt.ss.p.enable\tEnable filter supersampling. \nAllows to run the subsequent filters at a higher rate than the PI is running, because it counts the output of the PI multiple times as valid.\t\nflt.ss.p.rate\tThe decimation factor for supersampling. \nA sample is valid every time this counter is reached on the base clock (62.5MHz or 50MHz on the FlexRIO and 40MHz on the USB-RIO)\t\nflt.bypass\tBypasses (disables) each of the total of 8 second order sections.\t\nflt.p.anot\tSecond order section denominators in pairs of 2. Values need to be inverted before writing!\t\nflt.p.b\tSecond order section nominator values in pairs of 3.\t\nflt.o.height\tOutput height after filtering for user display and debugging, not for image display.\t\n\n\nlwr: Local wave recording\nName\tDescription\tLimit\nlwr.p.start\tStart recording cycle-indexed inputs for averaged saving to memory.\t\nlwr.p.avgCnt\tNumber of averages to record as power-of-two.\t\nlwr.p.readAddress\tCycle index of memory position to read the recorded average from\t\nlwr.o.readData\tReturn value from the address requested in readAddress\t\n\n\nse: Scan Engine\nName\tDescription\tLimit\nse.p.clocks\tSets all the speeds and decimation factors for the scan process.\tNot FlexRIO\nse.p.clocks->outputRate\tSets the IO sample rate of the scan waveform based on the base clock.\tNot FlexRIO\nse.p.clocks->fastDecFactor\tSets the ticks per step of the fast scan axis wave based on outputRate\tNot FlexRIO\nse.p.clocks->outWaveSizeFast\tThe total length of the fast axis drive waveform\tNot FlexRIO\nse.p.clocks->pplUpsampling\tSets the number of outputRate steps before a pixel is recorded\tNot FlexRIO\nse.p.clocks->numLines\tThis is the number of lines per image. This is used to reset the slow axis clocks\tNot FlexRIO\nse.p.clocks->se.p.fastInvDec\tInverse of fastDecFactor, calculated on host to ease resource usage on target\tNot FlexRIO\nse.p.clocks->se.p.slowUpStep\tIncremental step of the slow waveform for each outputRate cycle. \nThis sets the speed of the slow waveform\tNot FlexRIO\nse.p.clocks->se.p.outWaveSizeSlow\tTotal size of points of the slow scan direction waveform\tNot FlexRIO\nse.p.modes\tModal parameters of the scan process. \nenable starts the scanning. singleDirection returns the scan to the origin after one \"up\" frame without scanning back down. \nhaltScan can be used to temporarily interrupt the scan and stay in one place. \nse.mot.p.start starts a manual movement of the scan engine towards a target point (see se.mot for parameters)\tNot FlexRIO\nse.p.fastBlanking\tUsed for overscanning. \nThis gives the ranges of indexes of the fast scan waveform in which pixels are acquired, one for forward, \none for backward as well as a bypass\tNot FlexRIO\nse.p.scanSize\tThe size of the scanned area from 0 to 1, corresponding to no scan to full DAC range\tNot FlexRIO\nse.p.scanOffsets\tScan area offset from -1 to 1\tNot FlexRIO\nse.p.transformMatrix\tOutput matrix transformation, used for rotation and shear correction.\tNot FlexRIO\nse.m.fastAxis\tMemory access node for the fast scan direction waveform\tNot FlexRIO\nse.m.slowAxis\tMemory access node for the slow scan direction waveform\tNot FlexRIO\nse.s.ticksPerPixel\tStatus display for the real amount of ticks base clock that pass per pixel\tNot FlexRIO\nse.s.realXYOutputRate\tStatus display for the real amount of ticks base clock that pass per output point. \nShould correspond to the one set in se.clocks\tNot FlexRIO\n\n\nse.mot: Manual positioning of the tip in XY direction\nName\tDescription\tLimit\nse.mot.p.target\tTarget location to move to, in coordinates of -1 to 1\tNot FlexRIO\nse.mot.s.running\tIndicator wether the manual positioning is currently actively changing position\tNot FlexRIO\nse.mot.p.clocks\tSpeed settings for the manual positioning. \nmoveToDecFactor is clocked on the output rate and sets the decimation of how fast the movement is replayed. \nmoveToWaveSize is the number of points in the manual motion waveform. \ninvDec is the inverse of moveToDecFactor, computed on host for reduced resource usage.\tNot FlexRIO\nse.mot.m.motion\tMemory access node for the waveform that is replayed when moving manually \n(constant acceleration s-shape)\tNot FlexRIO\nse.mot.s.origin\tDebug indicator for the last saved origin before the motion is started.\tNot FlexRIO\nsmd: Stepper motor driver\n\nName\tDescription\tLimit\nsmd.p.address\tSteps the memory of the 4-value memory for all stepper motor coils\tNot FlexRIO\nsmd.m.writeMem\tMemory access node for the digital values that are sent to the stepper motor (usually half-step drive)\tNot FlexRIO\nitc: inter target communication\nort.bgc.requestType\tSets the request for background correction to the ORT engine. \nThis is typically used to force a background correction at the end of each frame.\tNot FlexRIO"
  # "Variables\n\ncomponent.[subcomponent.][imops.]element\n\ni: input\no: output\np: process\ns: status\nm: memory access\n\n\nRegisters and memory\ncomponent.element\n\n\nFIFOs\n\ncomponent[-destinationComponent].scope.element\n\nScopes:\nt: Target scoped\nth2: Target to Host\nh2t: Host to target\n\n\nAvailable components\n\naio: Analog in-output\ncls: Closed-loop scan\nfb: Feedback\nfb.mot Manual feedback motion\nfb.loff Lift-off system\nflt Digital signal filtering\nflt.ss Filter supersampling of input\nhdt: Image data transfer to host computer\nhdt.ort ORT data transfer\nhdt.aux Auxiliary channel data transfer\nhsdc: High-speed data capture, large volume raw input and corrected trace aquisition\nitc: Inter-target communication\nlwr: Local wave recording, aquire synchronously averaged cycle traces\nort: Off-resonance tapping\nort.fit: Real-time curve fitting\nort.bgc: Background correction\nsmd: Stepper motor drive\nse: Scan engine\nse.mot: Point target motion for scan enginese\nsid: System identification\n\n\nFPGA target types\n\nPXIE_7975R Kintex7 flexRIO, hsFeedback 250MSps\nPXI_7954R Virtex5 flexRIO, hsFeedback 100MSps\nPXI_7851R Virtex5 scanEngine for HS setup 750kSps\nPXI_7842R Virtex5 scanEngine for Hs setup 200kSps\nUSB_7856R_OEM Kintex7 All-in-one 1MSps\n\n\nIRQ Numbers\n\n4: background ready\n5: interaction start\n6: HSDC ready\n7: lwr ready"
  n1 = disable-structure shown="CTLR_PROVIDE_SCAN==1" {
    frame condition #0 {
    }
    frame condition #1 (active) {
      n2 = node-c288() -> (w2:T44)  [unwired: 1 in]
      n3 = while {
        stop <- FALSE stop-if-true
        # "Memory write access for scan engine"
        n4 = Unbundle By Name("se.m.slowAxis") -> ("write"=w79:bool, "index"=w81:u16, "data"=w80:fxp<+/-,18,2>)
        n5 = Unbundle By Name("se.m.fastAxis") -> ("write"=w77:bool, "index"=w76:u16, "data"=w75:fxp<+/-,18,2>)
        n6 = case shown="True" w79 {
          tunnel: w81 -> [_ w93]
          tunnel: w80 -> [_ w92]
          frame False {
          }
          frame True {
            n7 = xnode ("Memory Method Node")("Address"=w93, "Data"=w92) -> ()  [unwired: 1 in, 1 out]
          }
        }
        n8 = case shown="True" w77 {
          tunnel: w76 -> [_ w91]
          tunnel: w75 -> [_ w90]
          frame False {
          }
          frame True {
            n9 = xnode ("Memory Method Node")("Address"=w91, "Data"=w90) -> ()  [unwired: 1 in, 1 out]
          }
        }
        n10 = Unbundle By Name("se.mot.m.motion") -> ("write"=w73:bool, "index"=w71:u16, "data"=w72:fxp<+/-,18,1>)
        n11 = Unbundle By Name("smd.p.writeMem") -> ("write"=w68:bool, "index"=w69:u16, "data"=w70:bool[])
        n12 = case shown="True" w73 {
          tunnel: w72 -> [_ w89]
          tunnel: w71 -> [_ w88]
          frame False {
          }
          frame True {
            n13 = xnode ("Memory Method Node")("Address"=w88, "Data"=w89) -> ()  [unwired: 1 in, 1 out]
          }
        }
        n14 = case shown="True" w68 {
          tunnel: w70 -> [_ w87]
          tunnel: w69 -> [_ w86]
          frame False {
          }
          frame True {
            n15 = xnode ("Memory Method Node")("Address"=w86, "Data"=w87) -> ()  [unwired: 1 in, 1 out]
          }
        }
        n16 = Unbundle By Name("se.sid.prbs") -> ("write"=w64:bool, "index"=w66:u16, "data"=w65:bool)
        n17 = case shown="True" w64 {
          tunnel: w65 -> [_ w85]
          tunnel: w66 -> [_ w84]
          frame False {
          }
          frame True {
            n18 = xnode ("Memory Method Node")("Address"=w84, "Data"=w85) -> ()  [unwired: 1 in, 1 out]
          }
        }
      }
      n19 = timed-loop {
        timing: w2 -> [_]
        timing-out: [_] -> w1
        stop <- _ stop-if-true
        # "Add sensor input"
        # "scan loop"
        n20 = feedback #1() -> (w26:bool)  [unwired: 1 in]
        n21 = xnode ("FIFO Read Using Handshaking")("Ready for Output"=w26) -> ("Element"=w27:cluster{"a":i16, "b":i16}, "Output Valid"=w12:bool)  [unwired: 1 in, 1 out]
        n22 = Bundle("se.p.scanOffsets"="se.p.scanOffsets", "se.p.transformMatrix"="se.p.transformMatrix", "se.p.scanSize"="se.p.scanSize") -> (w48:T47)  [unwired: 1 in]
        n23 = Bundle("se.mot.p.clocks"="se.mot.p.clocks", "se.p.clocks"="se.p.clocks") -> (w49:T48)  [unwired: 1 in]
        n24 = case shown="True" "se.sid.start" {
          frame False {
          }
          frame True {
            n25 = local write "se.sid.start"(FALSE ("se.sid.start")) -> ()
          }
        }
        n26 = Unbundle(w27) -> ("a"=w14:i16, "b"=w13:i16)
        n27 = call "se_main.vi"("se.mot.p.target"="se.mot.p.target", "outputParams"=w48, "se.p.modes"="se.p.modes", "se.p.durationTrigger"="se.p.durationTrigger", "scanClocks"=w49) -> ("clocksOut"=→"clocksOut":T8, "se.o.position"=w40:T49, "se.mot.s.origin"=→"se.mot.s.origin":T50, "se.mot.s.running"=→"se.mot.s.running":bool, "se.s.blankingOff"=→"se.s.blankingOff":bool)  [unwired: 2 out]
        "se.o.position" <- w40
        n28 = Unbundle By Name("se.p.modes") -> ("se.mot.p.start"=w46:bool)
        n29 = call "se_sid_main.vi"("se.sid.start"="se.sid.start", "axisXNotY"="se.sid.p.axisXNotY", "sysIdParams"="se.sid.p.params", "se.sid.i.position"=w40) -> ("se.sid.s.repetitions"=→"se.sid.s.repetitions":u16, "se.sid.s.running"=→"se.sid.s.running":bool, "se.sid.o.position"=w39:T51)  [unwired: 4 in, 1 out]
        n30 = Bundle By Name(cluster="se.p.modes", "se.mot.p.start"=FALSE) -> (w43:T5)
        n31 = Unbundle(w39) -> ("outputInt"=w19:T52, w17:bool)
        n32 = feedback-in #2(w46) -> ()
        n33 = feedback #2() -> (w45:bool)  [unwired: 1 in]
        n34 = feedback-in #3(w19, w17) -> ()
        n35 = feedback #3() -> (w23:T52)  [unwired: 1 in]
        n36 = case shown="True" w45 {
          tunnel: w43 -> [_ w58]
          frame False {
          }
          frame True {
            n37 = local write "se.p.modes"(w58) -> ()
          }
        }
        n38 = Unbundle(w23) -> ("sid.o.height"=w25:fxp<+/-,28,1>, "sid.o.height"=w24:fxp<+/-,28,1>)
        n39 = Bundle By Name(cluster="se.p.x.fbParams", "setPoint"=w25) -> (w28:T9)
        n40 = Bundle By Name(cluster="se.p.y.fbParams", "setPoint"=w24) -> (w30:T9)
        n41 = call "pid_XY.vi"("inputValid"=w12, "fbParams"=w28, "input"=w14) -> ("output valid"=w15:bool, "output"=w21:T53, "ready for input"=w11:bool)  [unwired: 6 in]
        n42 = feedback-in #1(w11) -> ()
        n43 = call "pid_XY.vi"("inputValid"=w12, "fbParams"=w30, "input"=w13) -> ("output"=w22:T53)  [unwired: 6 in, 2 out]
        n44 = Unbundle(w21) -> ("X"=w10:fxp<+/-,28,1>)  [unwired: 2 out]
        n45 = Unbundle(w22) -> ("X"=w9:fxp<+/-,28,1>)  [unwired: 2 out]
        n46 = Bundle("X"=w10, "X"=w9) -> (w20:cluster{"X":fxp<+/-,28,1>, "X":fxp<+/-,28,1>})  [unwired: 1 in]
        n47 = Select(t=w15, s="se.p.closedLoop", f=w17) -> (s? t:f=w16:bool)
        n48 = Select(t=w20, s="se.p.closedLoop", f=w19) -> (s? t:f=w8:T52)
        n49 = Unbundle(w8) -> ("sid.o.height"=w4:fxp<+/-,28,1>, "sid.o.height"=w6:fxp<+/-,28,1>)
        n50 = xnode "Reinterpret Number"("x"=w4) -> ("y"=w3:fxp<+/-,28,16>)
        n51 = xnode "Reinterpret Number"("x"=w6) -> ("y"=w5:fxp<+/-,28,16>)
        n52 = Bundle("y"=w3, "y"=w5) -> (w7:cluster{"y":fxp<+/-,28,16>, "y":fxp<+/-,28,16>})  [unwired: 1 in]
        n53 = xnode ("FIFO Method Node")("Element"=w7, "Input Valid"=w16) -> ()  [unwired: 1 in, 2 out]
      }
      n54 = node-c288(w1) -> ()
    }
  }
  n55 = disable-structure shown="FPGA_TARGET_CLASS==PXIE_7975R" {
    frame condition #0 (active) {
    }
    frame condition #1 {
      # "Remove false on terminal of  ITC collect pixel"
      n56 = node-c288() -> (w102:T44)  [unwired: 1 in]
      n57 = timed-loop {
        timing: w102 -> [_]
        timing-out: [_] -> w101
        stop <- _ stop-if-true
        n58 = xnode ("Memory Method Node")("Ready for Output"=TRUE) -> ("Data"=w132:T32, "Output Valid"=w127:bool)  [unwired: 1 in, 1 out]
        n59 = feedback-in #4("hsdc.o.address") -> ()
        n60 = feedback #4() -> (w129:u32)  [unwired: 1 in]
        n61 = Not Equal?(x="hsdc.o.address", y=w129) -> (x != y?=w130:bool)
        n62 = xnode ("Memory Method Node")("Address"="hsdc.o.address", "Input Valid"=w130) -> ()  [unwired: 1 in, 2 out]
        n63 = feedback-in #5(w132, w127) -> ()
        n64 = feedback #5() -> (→"hsdc.o.read":T32)  [unwired: 1 in]
      }
      n65 = node-c288(w101) -> ()
      n66 = node-c288() -> (w96:T44)  [unwired: 1 in]
      n67 = while {
        stop <- FALSE stop-if-true
        # "HSDC recording and tranfer control"
        n68 = call "hsdc_hypervisor.vi"("hsdc.p.start"="hsdc.p.start") -> ()  [unwired: 11 in]
      }
      n69 = timed-loop {
        timing: w96 -> [_]
        timing-out: [_] -> w95
        stop <- _ stop-if-true
        n70 = call "itc_collect_auxPixelEvents.vi"() -> ()  [unwired: 12 in]
      }
      n71 = node-c288(w95) -> ()
      n72 = node-c288(refnum<k21> "62.5MHz" ("Source Name")) -> (w98:T44)
      n73 = node-c288() -> (w100:T44)  [unwired: 1 in]
      n74 = timed-loop {
        timing: w98 -> [_]
        timing-out: [_] -> w97
        stop <- _ stop-if-true
        n75 = xnode "FPGA I/O Node"() -> ("itc-hdt.clearPixel"=w109)  [unwired: 1 in, 1 out]
        n76 = call <instrlib>:"Detect Rising Edge.vi"("signal"=w109) -> ("edge detected"=w107:bool)  [unwired: 14 in]
        n77 = xnode ("FIFO Method Node")("Element"=TRUE, "Input Valid"=w107) -> ()  [unwired: 1 in, 2 out]
      }
      n78 = timed-loop {
        timing: w100 -> [_]
        timing-out: [_] -> w99
        stop <- _ stop-if-true
        n79 = xnode "FPGA I/O Node"() -> ("pixelSync"=w119)  [unwired: 1 in, 1 out]
        n80 = call <instrlib>:"Detect Rising Edge.vi"("signal"=w119) -> ("edge detected"=w118:bool)  [unwired: 14 in]
        n81 = case shown="True" w118 {
          frame False {
          }
          frame True {
            n82 = xnode ("FIFO Method Node")("Element"=FALSE, "Timeout"=0) -> ()  [unwired: 1 in, 2 out]
          }
        }
      }
      n83 = node-c288(w99) -> ()
      n84 = node-c288(w97) -> ()
    }
  }
  n85 = disable-structure shown="FPGA_TARGET_CLASS==PXI_7851R||FPGA_TARGET_CLASS==PXI_7841R" {
    frame condition #0 (active) {
    }
    frame condition #1 {
      n86 = node-c288() -> (w140:T44)  [unwired: 1 in]
      n87 = node-c288() -> (w138:T44)  [unwired: 1 in]
      n88 = timed-loop {
        timing: w140 -> [_]
        timing-out: [_] -> w139
        stop <- _ stop-if-true
        n89 = xnode "FPGA I/O Node"() -> ("pixelSyncAux"=w146)  [unwired: 1 in, 1 out]
        n90 = call <instrlib>:"Detect Rising Edge.vi"("signal"=w146) -> ("edge detected"=w145:bool)  [unwired: 14 in]
        n91 = case shown="True" w145 {
          frame False {
          }
          frame True {
            n92 = xnode ("FIFO Method Node")("Element"=FALSE, "Timeout"=0) -> ()  [unwired: 1 in, 2 out]
          }
        }
      }
      n93 = timed-loop {
        timing: w138 -> [_]
        timing-out: [_] -> w137
        stop <- _ stop-if-true
        n94 = call "itc_clearPixel.vi"() -> ()  [unwired: 12 in]
        n95 = call "itc_collect_pixelEvents_sctl.vi"() -> ()  [unwired: 12 in]
      }
      n96 = node-c288(w137) -> ()
      n97 = node-c288(w139) -> ()
    }
  }
  n98 = disable-structure shown="CTLR_PROVIDE_FB==1" {
    frame condition #0 (active) {
      n99 = disable-structure shown="FPGA_TARGET_CLASS==USB_7856R_OEM||FPGA_TARGET_CLASS==USB_7856R" {
        disable-tunnel: [refnum<k21> "62.5MHz" ("Source Name") refnum<k21> "62.5MHz" ("Source Name") refnum<k21> "50MHz" ("Source Name") refnum<k21> "40 MHz Onboard Clock" ("Source Name")] -> w153
        frame condition #0 {
        }
        frame condition #1 {
        }
        frame condition #2 {
        }
        frame condition #3 (active) {
        }
      }
      n100 = disable-structure shown="FPGA_TARGET_CLASS==USB_7856R_OEM" {
        disable-tunnel: [refnum<k21> "IO Module\\Data Clock" ("Source Name") refnum<k21> "40 MHz Onboard Clock" ("Source Name") refnum<k21> "160MHz" ("aio.s.clock") _] -> w161
        frame condition #0 {
        }
        frame condition #1 (active) {
        }
        frame condition #2 {
        }
        frame condition #3 {
        }
      }
      "aio.s.clock" <- w161
      n101 = node-c288() -> (w157:T44)  [unwired: 1 in]
      n102 = disable-structure shown="CTLR_PROVIDE_SICM==1" {
        disable-tunnel: w153 -> [w684 _]
        frame condition #0 (active) {
          n103 = node-c288(w684) -> (w686:T44)
          n104 = timed-loop {
            timing: w686 -> [_]
            timing-out: [_] -> w685
            stop <- _ stop-if-true
            # "SICM"
            n105 = xnode ("FIFO Method Node")("Ready for Output"=TRUE) -> ("Element"=w700:fxp<+/-,24,16>, "Output Valid"=w701:bool)  [unwired: 1 in, 1 out]
            n106 = Bundle("Element"=w700, "Output Valid"=w701) -> (w703:T56)  [unwired: 1 in]
            n107 = call "sicm_main.vi"("sicm.blc.p.params"="sicm.blc.p.params", "sicm.display"="sicm.display", "sicm.p.clocks"="sicm.p.clocks", "sicm.p.params"="sicm.p.params", "sicm.p.modes"="sicm.p.modes", "sicm.i.current"=w703) -> ("sicm.debug"=→"sicm.Debug":T57, "sicm.s.baseline"=→"sicm.s.baseline":T40, "sicm.triggerHeight"=w698:T58, "heightOut"=w699:T59)  [unwired: 2 in]
            n108 = Unbundle(w698) -> ("x-y"=w690:fxp<+/-,22,4>, "output valid"=w689:bool)
            n109 = Unbundle(w699) -> ("x+y"=w687:fxp<+/-,28,2>, "output valid"=w697:bool)
            n110 = feedback #6() -> (→"sicm-hdt.t.triggerHeight":fxp<+/-,22,4>)  [unwired: 1 in]
            n111 = feedback-in #6(w690, w689) -> ()
            n112 = feedback #7() -> (→"sicm.o.height":fxp<+/-,28,2>)  [unwired: 1 in]
            n113 = feedback-in #7(w687, w697) -> ()
            n114 = xnode ("FIFO Method Node")("Element"=w687, "Input Valid"=w697) -> ()  [unwired: 1 in, 2 out]
            n115 = xnode ("FIFO Method Node")("Element"=w690, "Input Valid"=w689) -> ()  [unwired: 1 in, 2 out]
          }
          n116 = node-c288(w685) -> ()
        }
        frame condition #1 {
        }
      }
      n117 = node-c288(refnum<k21> "40 MHz Onboard Clock" ("Source Name")) -> (w163:T44)
      n118 = node-c288(w153) -> (w159:T44)
      n119 = node-c288(w161) -> (w167:T44)
      n120 = node-c288(w153) -> (w165:T44)
      n121 = node-c288(w153) -> (w155:T44)
      n122 = timed-loop {
        timing: w157 -> [_]
        timing-out: [_] -> w156
        stop <- _ stop-if-true
        # "Host data averaging"
        n123 = call "hdt_main_averageChannels.vi"("outSteamSelect"="hdt.mainOutStreamSelect", "hdt.p.averageEnabled"="hdt.p.mainAverageEnabled", "enableOutput"="hdt.o.enable") -> ("debugStream"=→"hdt.debugStream":T22)  [unwired: 8 in]
      }
      n124 = timed-loop {
        timing: w163 -> [_]
        timing-out: [_] -> w162
        stop <- _ stop-if-true
        # "Slow fit calculations"
        n125 = call "ort_fit_calcSlopeDissipation.vi"() -> ()  [unwired: 11 in, 1 out]
      }
      n126 = timed-loop {
        timing: w159 -> [_]
        timing-out: [_] -> w158
        stop <- _ stop-if-true
        # "2 stages"
        # "Filters"
        # "Can be used to hold the output while filters are being enabled to prevent jumps from transients."
        # "Replace this with an actual external trigger line"
        # "Use this to implement direct feedback signal access (e.g SICM or ramp modes)"
        # "output supersampling"
        # "PID calculation and height control"
        n127 = feedback #8() -> (w414:bool)  [unwired: 1 in]
        n128 = xnode ("FIFO Method Node")("Ready for Output"=w414) -> ("Element"=w405:fxp<+/-,24,16>, "Output Valid"=w364:bool)  [unwired: 1 in, 1 out]
        n129 = feedback #9() -> (w404:fxp<+/-,24,16>)  [unwired: 1 in]
        "fb.i.raw" <- w404
        n130 = feedback-in #9(w405, w364) -> ()
        n131 = disable-structure shown="FPGA_TARGET_CLASS==USB_7856R_OEM||FPGA_TARGET_CLASS==USB_7856R" {
          disable-tunnel: [w426 w427 _] -> w396
          frame condition #0 {
            n132 = xnode "FPGA I/O Node"() -> ("switchForceSetpoint"=w426)  [unwired: 1 in, 1 out]
          }
          frame condition #1 (active) {
            n133 = xnode ("Register Read")() -> ("Data"=w427:bool)  [unwired: 1 in, 1 out]
          }
          frame condition #2 {
          }
        }
        n134 = disable-structure shown="CTLR_PROVIDE_SICM==1" {
          disable-tunnel: [w421 T55 {"Element"=0.0, "Output Valid"=FALSE}] -> w357
          frame condition #0 (active) {
            n135 = xnode ("FIFO Method Node")("Ready for Output"=TRUE) -> ("Element"=w423:fxp<+/-,22,4>, "Output Valid"=w422:bool)  [unwired: 1 in, 1 out]
            n136 = Bundle("Element"=w423, "Output Valid"=w422) -> (w421:T55)  [unwired: 1 in]
          }
          frame condition #1 {
          }
        }
        n137 = xnode "Reinterpret Number"("x"=w404) -> ("y"=w365:fxp<+/-,24,1>)
        "fb.i.rescaled" <- w365
        n138 = xnode ("Register Read")() -> ("Data"=w407:bool)  [unwired: 1 in, 1 out]
        n139 = Unbundle By Name("fb.p.params") -> ("setPointAlt"=w401:fxp<+/-,17,1>, "setPoint"=w402:fxp<+/-,17,1>, "pGain"=w399:fxp<+/-,20,4>, "iGain"=w398:fxp<+/-,20,1>, "gainScale"=w397:i8)
        n140 = Unbundle("fb.loff.p.params") -> ("liftHeight"=w409:fxp<+/-,15,4>, "disengagePos"=w408:fxp<+/-,22,1>)
        n141 = Compound Arithmetic op=AND("fb.p.allowSetpointSwitch", w396) -> (w394:bool)
        n142 = Bundle("y"=w365, "Output Valid"=w364) -> (w361:cluster{"y":fxp<+/-,24,1>, "Output Valid":bool})  [unwired: 1 in]
        n143 = Select(t=w401, s=w394, f=w402) -> (s? t:f=w400:fxp<+/-,17,1>)
        n144 = xnode ("Register Write")("Data"="fb.p.enable") -> ()  [unwired: 1 in, 1 out]
        n145 = Bundle By Name(cluster=T54 {"liftHeight"=0.0498046875, "disengagePos"=-1.0, "liftOff"=FALSE} ("liftOffParams"), "liftHeight"=w409, "disengagePos"=w408, "liftOff"=w407) -> (w406:T54)
        n146 = Bundle By Name(cluster=T9 {"enable"=FALSE, "setPoint"=0.001007080078125, "pGain"=0.0, "iGain"=0.10000038146972656, "gainScale"=0} ("fbParams"), "enable"="fb.p.enable", "setPoint"=w400, "pGain"=w399, "iGain"=w398, "gainScale"=w397) -> (w392:T9)
        n147 = Bundle By Name(cluster="fb.mot.p.params", "doMove"=FALSE) -> (w386:T27)
        n148 = Unbundle By Name("fb.mot.p.params") -> ("doMove"=w322:bool)
        n149 = case shown="True" w322 {
          tunnel: w386 -> [_ w425]
          frame False {
          }
          frame True {
            n150 = local write "fb.mot.p.params"(w425) -> ()
          }
        }
        n151 = feedback #10() -> (w345:fxp<+/-,31,4>)  [unwired: 1 in]
        n152 = Bundle By Name(cluster="rmp.p.params", "rmp.p.startPos"=w345) -> (w349:T41)
        n153 = feedback #11() -> (w367:bool)  [unwired: 1 in]
        n154 = call "pid_main_v2.vi"("limits"="fb.p.limits", "ready for output (T)"=w367, "manualMotion"="fb.mot.p.params", "inputValid"=w364, "liftOffParams"=w406, "fbParams"=w392, "input"=w405) -> ("output valid"=w340:bool, "output"=w412:T60, "ready for input"=w413:bool)  [unwired: 2 in]
        n155 = feedback-in #8(w413) -> ()
        n156 = Unbundle By Name(w412) -> ("zHeight"=w369:fxp<+/-,28,1>, "error"=w332:fxp<+/-,25,2>, "pidAtLimit"=→"fb.s.atLimit":bool, "moving"=w390:bool)  [unwired: 1 out]
        "fb.mot.s.running" <- w390
        n157 = xnode ("FIFO Method Node")("Element"=w332, "Input Valid"=w340) -> ()  [unwired: 1 in, 2 out]
        n158 = xnode ("Register Write")("Data"=w390) -> ()  [unwired: 1 in, 1 out]
        n159 = case shown="True" "sid.p.start" {
          frame False {
          }
          frame True {
            n160 = local write "sid.p.start"(FALSE ("sid.p.start")) -> ()
          }
        }
        n161 = feedback #12() -> (w354:bool)  [unwired: 1 in]
        n162 = xnode ("Register Write")("Data"=w354) -> ()  [unwired: 1 in, 1 out]
        n163 = Unbundle By Name("rmp.p.action") -> ("rmp.p.start"=w319:bool)
        n164 = Select(t=w349, s="rmp.p.useIntHeightAsStart", f="rmp.p.params") -> (s? t:f=w348:T41)
        n165 = feedback #13() -> (w352:T61)  [unwired: 1 in]
        n166 = Build Array(w361, w357, w352) -> (w360:T62)
        n167 = Index Array(array=w360, index="flt.i.bypassSource") -> (element=w358:T63)
        n168 = Unbundle(w358) -> ("Element"=w363:fxp<+/-,27,4>, "rmp.o.valid"=w362:bool)
        n169 = Select(t=w363, s="flt.bypassPI", f=w369) -> (s? t:f=w331:fxp<+/-,31,4>)
        "fb.o.height" <- w331
        n170 = Select(t=w362, s="flt.bypassPI", f=w340) -> (s? t:f=w333:bool)
        n171 = Bundle("error"=w332, "output valid"=w333) -> (w335:T64)  [unwired: 1 in]
        n172 = Bundle("zHeight"=w331, "output valid"=w333) -> (w334:T65)  [unwired: 1 in]
        n173 = feedback-in #10(w331, w333) -> ()
        n174 = Build Array(w335, w334) -> (w336:T66)
        n175 = xnode ("FIFO Method Node")("Element"=w331, "Input Valid"=w333) -> ()  [unwired: 1 in, 2 out]
        n176 = Index Array(array=w336, index="sid.p.idSource") -> (element=w330:T65)
        n177 = Greater?(x=w331, y="fb.p.zWatchDogTreshold") -> (0:w355:bool)
        n178 = call "sid_main.vi"("idVar"=w330, "sid.allowExternalRecord"="sid.allowExternalRecord", "inputValid"=w333, "sid.p.params"="sid.p.params", "sid.p.start"="sid.p.start", "sid.i.height"=w331) -> ("outputValid"=w342:bool, "sid.running"=→"sid.s.running":bool, "sid.o.height"=w341:fxp<+/-,43,16>, "sid.o.count"=→"sid.o.count":u16)  [unwired: 1 in, 1 out]
        n179 = feedback-in #12(w355, w333) -> ()
        n180 = call "rmp_main.vi"("rmp.i.externalTrigger"=FALSE, "rmp.p.reset"="rmp.p.reset", "rmp.p.action"="rmp.p.action", "rmp.p.triggerParams"="rmp.p.triggerParams", "rmp.p.params"=w348) -> ("rmp.s.running"=→"rmp.s.running":bool, "rmp.o.height"=w353:T61)  [unwired: 5 in]
        n181 = feedback-in #13(w353) -> ()
        n182 = case shown="True" w319 {
          tunnel: "rmp.p.action" -> [_ w418]
          frame False {
          }
          frame True {
            n183 = Bundle By Name(cluster=w418, "rmp.p.start"=FALSE ("rmp.i.externalTrigger")) -> (w419:cluster{"rmp.p.start":bool, "rmp.p.stop":bool})
            n184 = local write "rmp.p.action"(w419) -> ()
          }
        }
        n185 = case shown="True" w319 {
          frame False {
          }
          frame True {
            n186 = local write "rmp.p.reset"(T43 {"rmp.p.resetStartPos"=FALSE, "rmp.p.resetEndPos"=FALSE} ("rmp.p.reset")) -> ()
          }
        }
        n187 = call "flt_sos8xblock.vi"("sosBypass"="flt.bypass1", "input valid"=w342, "b"="flt.p.b8x", "anot"="flt.p.anot8x", "input"=w341) -> ("output valid"=w371:bool, "output"=w377:fxp<+/-,20,2>)  [unwired: 4 in, 1 out]
        n188 = call "circularCounter_v2.vi"("reset"=w371, "maxCount"="flt.ss.p.rate") -> ("maxReached"=w383:bool)  [unwired: 6 in, 3 out]
        n189 = feedback #14() -> (w372:fxp<+/-,20,2>)  [unwired: 1 in]
        n190 = feedback-in #14(w377, w371) -> ()
        n191 = And(x=w383, y="flt.ss.p.enable") -> (x .and. y?=w381:bool)
        n192 = Or(x=w381, y=w371) -> (x .or. y?=w375:bool)
        n193 = call "flt_sos4xblock.vi"("sosBypass"="flt.bypass2", "input valid"=w375, "b"="flt.p.b4x", "anot"="flt.p.anot4x", "input"=w372) -> ("ready for input"=w368:bool, "output valid"=w327:bool, "output"=w325:fxp<+/-,20,2>)  [unwired: 4 in]
        "flt.o.height" <- w325
        n194 = feedback-in #11(w368) -> ()
        n195 = Compound Arithmetic op=AND(w327, invert "flt.o.hold") -> (w324:bool)
        n196 = feedback-in #15(w325, w324) -> ()
        n197 = feedback #15() -> (w328:fxp<+/-,20,2>)  [unwired: 1 in]
        n198 = xnode "Reinterpret Number"("x"=w328) -> ("y"=w385:fxp<+/-,20,17>)
        n199 = feedback-in #16(w327) -> ()
        n200 = feedback #16() -> (w326:bool)  [unwired: 1 in]
        n201 = To Fixed-Point(number=w385) -> (fixed-point=w366:fxp<+/-,18,16>)  [unwired: 1 in]
        n202 = xnode ("FIFO Method Node")("Element"=w366, "Input Valid"=w326) -> ()  [unwired: 1 in, 2 out]
      }
      n203 = timed-loop {
        timing: w167 -> [_]
        timing-out: [_] -> w166
        stop <- _ stop-if-true
        # "DO NOT PUT ANY CONTROLS OR INDICATORS INTO THIS LOOP. DOING SO WILL CRASH LABVIEW IN A CATASTROPHIC FASHION"
        # "Loop clocked by the IO"
        # "Vertical"
        # "Horiz"
        # "Input module aquisition and excitation output"
        n204 = disable-structure shown="FPGA_TARGET_CLASS==USB_7856R_OEM||FPGA_TARGET_CLASS==USB_7856R" {
          disable-tunnel: [w618 w636 i16 0 ("IO Module\\AI 1")] -> w563
          disable-tunnel: [w608 w622 _] -> w565
          disable-tunnel: [w617 w637 _] -> w564
          disable-tunnel: FALSE ("aio.i.zeroDeflection") -> [w619 w635 _]
          disable-tunnel: 1 ("index") -> [w613 w634 _]
          disable-tunnel: 0 ("index") -> [w614 w633 _]
          disable-tunnel: [w608 w624 _] -> w553
          frame condition #0 {
            n205 = xnode "FPGA I/O Node"() -> ("IO Module\\AI 0"=w616, "IO Module\\AI 1"=w615)  [unwired: 2 in, 2 out]
            n206 = xnode ("Register Read")() -> ("Data"=w610:bool[])  [unwired: 1 in, 1 out]
            n207 = call "circularCounter_v2.vi"("maxCount"=u16 4) -> ("maxPulse"=w621:bool)  [unwired: 7 in, 3 out]
            n208 = feedback #17() -> (w609:bool)  [unwired: 1 in]
            n209 = feedback-in #17(w621) -> ()
            n210 = Index Array(array=w610, index #1=w614, index #2=w613) -> (element #1=w612:bool, element #2=w611:bool)
            n211 = call "decimateInput.vi"("reset"=w609, "input"=w616, "zeroOutput"=w619, "invert"=w612) -> ("output"=w617:i16)  [unwired: 7 in]
            n212 = call "decimateInput.vi"("reset"=w609, "input"=w615, "zeroOutput"=w619, "invert"=w611) -> ("output"=w618:i16)  [unwired: 7 in]
            n213 = feedback-in #18(w609) -> ()
            n214 = feedback #18() -> (w608:bool)  [unwired: 1 in]
          }
          frame condition #1 (active) {
            w629 = TRUE ("Ready for Output")
            n215 = xnode ("FIFO Method Node")("Ready for Output"=w629) -> ("Element"=w639:cluster{"a":i16, "b":i16}, "Output Valid"=w622:bool)  [unwired: 1 in, 1 out]
            n216 = xnode ("Register Read")() -> ("Data"=w630:bool[])  [unwired: 1 in, 1 out]
            n217 = xnode ("Register Read")() -> ("Data"=w625:bool)  [unwired: 1 in, 1 out]
            n218 = xnode ("FIFO Method Node")("Ready for Output"=w629) -> ("Element"=w628:i16, "Output Valid"=w623:bool)  [unwired: 1 in, 1 out]
            n219 = Unbundle(w639) -> ("a"=w627:i16, "b"=w638:i16)
            n220 = Select(t=w628, s=w625, f=w627) -> (s? t:f=w626:i16)
            n221 = Select(t=w623, s=w625, f=w622) -> (s? t:f=w624:bool)
            n222 = Index Array(array=w630, index #1=w633, index #2=w634) -> (element #1=w632:bool, element #2=w631:bool)
            n223 = call "invert_and_blank_caseStruct.vi"("zeroOutput"=w635, "invert"=w631, "input"=w638) -> ("output"=w636:i16)  [unwired: 8 in]
            n224 = call "invert_and_blank_caseStruct.vi"("zeroOutput"=w635, "invert"=w632, "input"=w626) -> ("output"=w637:i16)  [unwired: 8 in]
          }
          frame condition #2 {
            w641 = i16 0 ("IO Module\\AI 0")
          }
        }
        n225 = xnode ("Register Read")() -> ("Data"=w570:u16)  [unwired: 1 in, 1 out]
        n226 = call "circularCounter_v2.vi"("doStep"=w553, "maxCount"=w570) -> ("maxReached"=w585:bool, "index"=w572:u16)  [unwired: 6 in, 2 out]
        n227 = xnode ("FIFO Method Node")("Element"=w563, "Input Valid"=w565) -> ()  [unwired: 1 in, 2 out]
        n228 = xnode ("FIFO Method Node")("Ready for Output"=TRUE) -> ("Element"=w583:fxp<+/-,18,16>, "Output Valid"=w584:bool)  [unwired: 1 in, 1 out]
        n229 = feedback-in #19(w572) -> ()
        n230 = feedback #19() -> (w575:u16)  [unwired: 1 in]
        n231 = feedback-in #20(w585) -> ()
        n232 = feedback #20() -> (w574:bool)  [unwired: 1 in]
        n233 = call <instrlib>:"Detect Falling Edge.vi"("signal"=w574) -> ("edge detected"=w573:bool)  [unwired: 14 in]
        n234 = Bundle By Name(cluster=cluster{"index":u16, "data":i16} {"index"=0, "data"=0} ("dataPair"), "index"=w575, "data"=w564) -> (w586:cluster{"index":u16, "data":i16})
        n235 = xnode ("Memory Method Node")("Address"=w575) -> ("Data"=w587:i16)  [unwired: 1 in, 1 out]
        n236 = xnode ("Handshake Write")("Data"=TRUE, "Input Valid"=w573) -> ()  [unwired: 1 in, 2 out]
        n237 = xnode ("FIFO Method Node")("Element"=w586, "Input Valid"=w553) -> ()  [unwired: 1 in, 2 out]
        n238 = feedback-in #21(w583, w584) -> ()
        n239 = feedback #21() -> (w554:fxp<+/-,18,16>)  [unwired: 1 in]
        n240 = feedback-in #22(w554) -> ()
        n241 = feedback #22() -> (w579:fxp<+/-,18,16>)  [unwired: 1 in]
        n242 = xnode ("Register Read")() -> ("Data"=w557:bool)  [unwired: 1 in, 1 out]
        n243 = feedback #23() -> (w567:i16)  [unwired: 1 in]
        n244 = feedback-in #23(w587) -> ()
        n245 = Select(t=i16 0, s=w557, f=w567) -> (s? t:f=w566:i16)
        n246 = To Fixed-Point(number=w566) -> (fixed-point=w578:fxp<+/-,16,16>)  [unwired: 1 in]
        n247 = xnode ("Register Read")() -> ("Data"=w556:bool)  [unwired: 1 in, 1 out]
        n248 = feedback-in #24(w578) -> ()
        n249 = feedback #24() -> (w576:fxp<+/-,16,16>)  [unwired: 1 in]
        n250 = xnode ("High Throughput Add")("x"=w576, "y"=w579) -> ("x+y"=w577:fxp<+/-,18,16>)
        n251 = xnode ("Register Read")() -> ("Data"=w555:bool)  [unwired: 1 in, 1 out]
        n252 = Select(t=w577, s=w556, f=w579) -> (s? t:f=w580:fxp<+/-,18,16>)
        n253 = xnode ("Register Read")() -> ("Data"=w550:cluster{"a":i16, "b":i16})  [unwired: 1 in, 1 out]
        n254 = Compound Arithmetic op=OR(w557, w556) -> (w571:bool)
        n255 = feedback-in #25(w580) -> ()
        n256 = feedback #25() -> (w559:fxp<+/-,18,16>)  [unwired: 1 in]
        n257 = Select(t=i16 0, s=w571, f=w567) -> (s? t:f=w569:i16)
        n258 = Negate(x=w559) -> (-x=w558:fxp<+/-,19,17>)
        n259 = Select(t=w559, s=w555, f=w558) -> (s? t:f=w552:fxp<+/-,19,17>)
        n260 = Unbundle(w550) -> ("a"=w549:i16, "b"=w548:i16)
        n261 = In Range and Coerce(upper limit=w549, x=w552, lower limit=w548) -> (coerced(x)=w551:fxp<+/-,19,17>)  [unwired: 1 out]
        n262 = disable-structure shown="FPGA_TARGET_CLASS==USB_7856R_OEM||FPGA_TARGET_CLASS==USB_7856R" {
          disable-tunnel: w551 -> [w593 w606 _]
          disable-tunnel: w569 -> [w592 w603 _]
          disable-tunnel: w565 -> [_ w604 _]
          disable-tunnel: w553 -> [_ w601 _]
          frame condition #0 {
            n263 = xnode ("Register Read")() -> ("Data"=w591:bool)  [unwired: 1 in, 1 out]
            n264 = xnode "FPGA I/O Node"("IO Module\\AO 0 N"=w592, "IO Module\\AO 0 N-1"=w592) -> ()  [unwired: 2 in, 2 out]
            n265 = feedback-in #26(w593) -> ()
            n266 = feedback #26() -> (w590:fxp<+/-,19,17>)  [unwired: 1 in]
            n267 = Bundle(cluster=cluster{i16, i16} {0, 0} ("s? t:f"), w590, w590) -> (w595:cluster{i16, i16})
            n268 = call "dither18bitTo16bit.vi"("input"=w590) -> ("output"=w599:cluster{i16, i16})  [unwired: 10 in]
            n269 = Select(t=w595, s=w591, f=w599) -> (s? t:f=w596:cluster{i16, i16})
            n270 = Unbundle(w596) -> (w598:i16, w597:i16)
            n271 = xnode "FPGA I/O Node"("IO Module\\AO 1 N-1"=w598, "IO Module\\AO 1 N"=w597) -> ()  [unwired: 2 in, 2 out]
          }
          frame condition #1 (active) {
            n272 = feedback-in #27(w606) -> ()
            n273 = feedback #27() -> (w600:fxp<+/-,19,17>)  [unwired: 1 in]
            n274 = To Word Integer(number=w600) -> (16bit integer=w605:i16)
            n275 = Bundle(w605, "Data"=w603) -> (w607:cluster{i16, "Data":i16})  [unwired: 1 in]
            n276 = feedback-in #28(w604) -> ()
            n277 = feedback #28() -> (w602:bool)  [unwired: 1 in]
            n278 = xnode ("FIFO Method Node")("Element"=w607, "Input Valid"=w602) -> ()  [unwired: 1 in, 2 out]
            n279 = xnode ("FIFO Method Node")("Element"=w603, "Input Valid"=w601) -> ()  [unwired: 1 in, 2 out]
          }
          frame condition #2 {
          }
        }
      }
      n280 = timed-loop {
        timing: w165 -> [_]
        timing-out: [_] -> w164
        stop <- _ stop-if-true
        # "Low pass filter\nadded for PORT"
        # "Auxiliary"
        # "Contact"
        # "ORT"
        # "Cycle-indexed value pairs"
        # "Main process variable calculation"
        n281 = xnode ("FIFO Method Node")("Ready for Output"=TRUE) -> ("Output Valid"=w527:bool)  [unwired: 1 in, 2 out]
        n282 = xnode ("FIFO Method Node")("Ready for Output"=TRUE) -> ("Element"=w475:cluster{"index":u16, "data":i16}, "Output Valid"=w470:bool)  [unwired: 1 in, 1 out]
        n283 = xnode ("Handshake Read")("Ready for Output"=TRUE) -> ("Output Valid"=w495:bool)  [unwired: 1 in, 2 out]
        n284 = xnode ("Register Write")("Data"="ort.p.waveSize") -> ()  [unwired: 1 in, 1 out]
        n285 = call "inputFilter_aio.vi"("Element in"=w475, "Output Valid"=w470, "aio.flt.p.b4x"="aio.flt.p.b4x", "aio.flt.p.anot4x"="aio.flt.p.anot4x", "aio.flt.bypass"="aio.flt.bypass") -> ("output valid"=w474:bool, "Element out"=w471:cluster{"index":u16, "y":fxp<+/-,20,17>})  [unwired: 5 in]
        n286 = xnode ("FIFO Method Node")("Ready for Output"=TRUE) -> ("Element"=w518:i16, "Output Valid"=w519:bool)  [unwired: 1 in, 1 out]
        n287 = Unbundle By Name(w471) -> ("y"=w477:fxp<+/-,20,17>)  [unwired: 1 out]
        "aio.s.fastVertical" <- w477
        n288 = feedback #29() -> (w505:fxp<+/-,20,17>)  [unwired: 1 in]
        n289 = feedback-in #29(w477, w474) -> ()
        n290 = call "ort_bgc_main.vi"("ort.bgc.p.bgCntP2"="ort.bgc.p.bgCntP2", "inputValid"=w474, "Data"=w471, "endOfWave"=w495) -> ("background"=w488:i16, "output"=w531:cluster{"index":u16, "data":i16}, "outptValid"=w487:bool)  [unwired: 5 in]
        "aio.s.ortSubstDeflection" <- w531
        n291 = To Fixed-Point(number=w505) -> (fixed-point=w503:fxp<+/-,24,16>)  [unwired: 1 in]
        n292 = xnode ("FIFO Method Node")("Element"=w518, "Input Valid"=w519) -> ()  [unwired: 1 in, 2 out]
        n293 = feedback #30() -> (w476:i16)  [unwired: 1 in]
        "aio.s.fastHoriz" <- w476
        n294 = feedback-in #30(w518, w519) -> ()
        n295 = call "lwr_main.vi"("inputValid"=w474, "readAddress"="lwr.p.readAddress", "endOfWave"=w495, "startRecording"=w527, "satCntP2"="lwr.p.avgCnt", "input"=w531) -> ("recordReady"=w522:bool, "readData"=→"lwr.o.readData":i32)  [unwired: 3 in, 1 out]
        n296 = To Fixed-Point(number=w476) -> (fixed-point=w511:fxp<+/-,24,16>)  [unwired: 1 in]
        "aio.s.HSaux" <- w511
        n297 = call <instrlib>:"Detect Rising Edge.vi"("signal"=w522) -> ("edge detected"=w521:bool)  [unwired: 14 in]
        n298 = call "ort_find_max.vi"("inputValid"=w487, "endOfCycle"=w495, "ort.p.methodParams"="ort.p.methodParams", "data"=w531) -> ("outputValid"=w504:bool, "cycleMaxMonitor"=→"ort.o.interactionMax":fxp<+/-,24,16>, "maxIndex"=→"ort.o.maxIndex":u16, "cycleMax"=w512:fxp<+/-,24,16>)  [unwired: 4 in]
        n299 = xnode ("FIFO Method Node")("Element"=TRUE, "Input Valid"=w521) -> ()  [unwired: 1 in, 2 out]
        n300 = call "ort_fit_start.vi"("inputValid"=w487, "ort.fit.p.params"="ort.fit.p.params", "data"=w531) -> ()  [unwired: 9 in]
        n301 = call "ort_fit_calcIntermediate.vi"("inputValid"=w474, "ort.fit.p.params"="ort.fit.p.params") -> ()  [unwired: 8 in, 2 out]
        n302 = Unbundle By Name(w531) -> ("index"=w490:u16, "data"=w489:i16)
        n303 = call "circularCounter_v2.vi"("doStep"=w474, "maxCount"="aio.i.samplingDecimation") -> ("maxPulse"=w500:bool)  [unwired: 6 in, 3 out]
        n304 = Bundle("index"=w490, "data"=w489, "background"=w488, "outptValid"=w487) -> (w486:T67)  [unwired: 1 in]
        n305 = disable-structure shown="FPGA_TARGET_CLASS==PXIE_7975R" {
          disable-tunnel: w487 -> [w538 _]
          disable-tunnel: w471 -> [w537 _]
          disable-tunnel: w474 -> [w536 _]
          disable-tunnel: w489 -> [w535 _]
          frame condition #0 {
            n306 = call "hsdc_record.vi"("hsdc.o.points"="hsdc.p.points", "hsdc.p.substBgnd"="hsdc.p.substBgnd", "subtractedValid"=w538, "subtracted"=w535, "rawValid"=w536, "raw"=w537) -> ()  [unwired: 6 in]
          }
          frame condition #1 (active) {
          }
        }
        n307 = feedback-in #31(w486) -> ()
        n308 = feedback #31() -> (w478:T67)  [unwired: 1 in]
        n309 = Bundle(w503, "maxPulse"=w500) -> (w502:cluster{fxp<+/-,24,16>, "maxPulse":bool})  [unwired: 1 in]
        n310 = Bundle("cycleMax"=w512, "outputValid"=w504) -> (w509:T68)  [unwired: 1 in]
        n311 = Bundle(w511, "maxPulse"=w500) -> (w510:cluster{fxp<+/-,24,16>, "maxPulse":bool})  [unwired: 1 in]
        n312 = call "intWaveMA.vi"("expFactor"="ort.p.fcAvg", "ortInput"=w478) -> ("ortOutput"=w493:T69)  [unwired: 8 in, 1 out]
        n313 = Build Array(w502, w509, w510) -> (w508:T70)
        n314 = Index Array(array=w508, index="fb.i.source") -> (element=w506:T71)
        n315 = Select(t=w493, s="ort.p.fcAvgEnable", f=w478) -> (s? t:f=w492:T67)
        n316 = feedback-in #32(w492) -> ()
        n317 = feedback #32() -> (w479:T69)  [unwired: 1 in]
        n318 = Unbundle(w506) -> ("cycleMax"=w499:fxp<+/-,24,16>, "maxPulse"=w498:bool)
        n319 = Unbundle(w479) -> ("index"=w483:u16, "data"=w482:i16, "background"=w491:i16, "inElementValid"=w481:bool)
        n320 = disable-structure shown="CTLR_PROVIDE_SICM==1" {
          disable-tunnel: w499 -> [w534 _]
          disable-tunnel: w498 -> [w533 _]
          frame condition #0 (active) {
            n321 = xnode ("FIFO Method Node")("Element"=w534, "Input Valid"=w533) -> ()  [unwired: 1 in, 2 out]
          }
          frame condition #1 {
          }
        }
        n322 = xnode ("FIFO Method Node")("Element"=w499, "Input Valid"=w498) -> ()  [unwired: 1 in, 2 out]
        n323 = Bundle("data"=w482, "background"=w491) -> (w494:cluster{"data":i16, "background":i16})  [unwired: 1 in]
        n324 = case shown="True" w481 {
          tunnel: w483 -> [_ w542]
          tunnel: w482 -> [_ w541]
          frame False {
          }
          frame True {
            n325 = xnode ("Memory Method Node")("Address"=w542, "Data"=w541) -> ()  [unwired: 1 in, 1 out]
            n326 = xnode ("Memory Method Node")("Address"=w542, "Data"=w541) -> ()  [unwired: 1 in, 1 out]
          }
        }
        n327 = Bundle("index"=w483, w494) -> (w480:T72)  [unwired: 1 in]
        n328 = xnode ("Handshake Write")("Data"=u16 0, "Input Valid"=w495) -> ()  [unwired: 1 in, 2 out]
        n329 = xnode ("FIFO Method Node")("Element"=w480, "Input Valid"=w481) -> ()  [unwired: 1 in, 2 out]
        n330 = xnode ("FIFO Method Node")("Element"=w499, "Input Valid"=w498) -> ()  [unwired: 1 in, 2 out]
        n331 = xnode ("FIFO Method Node")("Element"=w499, "Input Valid"=w498) -> ()  [unwired: 1 in, 2 out]
      }
      n332 = timed-loop {
        timing: w155 -> [_]
        timing-out: [_] -> w154
        stop <- _ stop-if-true
        # "Host data transfer interaction wave generator and memory control"
        n333 = Bundle By Name(cluster="hdt.int.p.readParams", "hdt.int.p.startTransfer"=FALSE) -> (w292:T21)
        n334 = Unbundle By Name("hdt.int.p.readParams") -> ("hdt.int.p.startTransfer"=w294:bool)
        n335 = call "hdt_int_generator.vi"("hdt.int.p.readParams"="hdt.int.p.readParams", "hdt.int.p.memWriteSource"="hdt.int.p.memWriteSource") -> ("hdt.int.s.debug"=→"hdt.int.s.debug":T20)  [unwired: 9 in]
        n336 = feedback-in #33(w294) -> ()
        n337 = feedback #33() -> (w291:bool)  [unwired: 1 in]
        n338 = case shown="True" w291 {
          tunnel: w292 -> [_ w295]
          frame False {
          }
          frame True {
            n339 = local write "hdt.int.p.readParams"(w295) -> ()
          }
        }
      }
      n340 = node-c288(w162) -> ()
      n341 = while {
        stop <- FALSE stop-if-true
        n342 = xnode ("Register Write")("Data"="aio.o.invertOutputs") -> ()  [unwired: 1 in, 1 out]
        n343 = xnode ("Register Read")("Data"="aio.o.invertInputs") -> ()  [unwired: 1 in, 1 out]
        n344 = xnode ("Register Read")("Data"="aio.o.invertHeight") -> ()  [unwired: 1 in, 1 out]
        n345 = xnode ("Register Read")("Data"="aio.o.invert2Inputs") -> ()  [unwired: 1 in, 1 out]
        n346 = xnode ("Register Read")("Data"="ort.o.piezoMode") -> ()  [unwired: 1 in, 1 out]
        n347 = xnode ("Register Read")("Data"="aio.o.disableExc") -> ()  [unwired: 1 in, 1 out]
        n348 = xnode ("Register Read")("Data"="aio.o.bypassDither") -> ()  [unwired: 1 in, 1 out]
        n349 = xnode ("Register Read")("Data"="aio.o.fastInput") -> ()  [unwired: 1 in, 1 out]
        n350 = disable-structure shown="FPGA_TARGET_CLASS==USB_7856R_OEM||FPGA_TARGET_CLASS==USB_7856R" {
          frame condition #0 (active) {
            n351 = disable-structure shown="FPGA_TARGET_CLASS==USB_7856R_OEM, Default" {
              disable-tunnel: "AI.voltage Range" -> [w744 w745]
              frame condition #0 {
                n352 = xnode "FPGA I/O Property Node"("Voltage Range"=w744) -> ()  [unwired: 1 in, 1 out]
                n353 = xnode "FPGA I/O Property Node"("Voltage Range"=w744) -> ()  [unwired: 1 in, 1 out]
                n354 = xnode "FPGA I/O Property Node"("Voltage Range"=w744) -> ()  [unwired: 1 in, 1 out]
                n355 = xnode "FPGA I/O Property Node"("Voltage Range"=w744) -> ()  [unwired: 1 in, 1 out]
                n356 = xnode "FPGA I/O Property Node"("Voltage Range"=w744) -> ()  [unwired: 1 in, 1 out]
                n357 = xnode "FPGA I/O Property Node"("Voltage Range"=w744) -> ()  [unwired: 1 in, 1 out]
                n358 = xnode "FPGA I/O Property Node"("Voltage Range"=w744) -> ()  [unwired: 1 in, 1 out]
                n359 = xnode "FPGA I/O Property Node"("Voltage Range"=w744) -> ()  [unwired: 1 in, 1 out]
              }
              frame condition #1 (active) {
                n360 = xnode "FPGA I/O Property Node"("Voltage Range"=w745) -> ()  [unwired: 1 in, 1 out]
                n361 = xnode "FPGA I/O Property Node"("Voltage Range"=w745) -> ()  [unwired: 1 in, 1 out]
                n362 = xnode "FPGA I/O Property Node"("Voltage Range"=w745) -> ()  [unwired: 1 in, 1 out]
                n363 = xnode "FPGA I/O Property Node"("Voltage Range"=w745) -> ()  [unwired: 1 in, 1 out]
                n364 = xnode "FPGA I/O Property Node"("Voltage Range"=w745) -> ()  [unwired: 1 in, 1 out]
                n365 = xnode "FPGA I/O Property Node"("Voltage Range"=w745) -> ()  [unwired: 1 in, 1 out]
                n366 = xnode "FPGA I/O Property Node"("Voltage Range"=w745) -> ()  [unwired: 1 in, 1 out]
                n367 = xnode "FPGA I/O Property Node"("Voltage Range"=w745) -> ()  [unwired: 1 in, 1 out]
              }
            }
          }
          frame condition #1 {
          }
        }
        n368 = xnode ("Register Read")("Data"="aio.o.heightLimits") -> ()  [unwired: 1 in, 1 out]
      }
      n369 = node-c288(w156) -> ()
      n370 = while {
        stop <- FALSE stop-if-true
        # "Host data transfer main"
        n371 = xnode ("FIFO Method Node")("Timeout"=-1) -> ("Element"=w750:fxp<+/-,22,1>[])  [unwired: 1 in, 2 out]
        n372 = for {
          tunnel: w750 -> [w753] mode=indexing
          n373 = xnode ("FIFO Method Node")("Element"=w753, "Timeout"=0) -> ("Timed Out?"=→"hdt.o.overflow":bool)  [unwired: 1 in, 1 out]
        }
        n374 = call "Tick Count"() -> ("Tick Count(Ticks)"=w747:u32)
        n375 = feedback #34() -> (w748:u32)  [unwired: 1 in]
        n376 = feedback-in #34(w747) -> ()
        n377 = Subtract(x=w747, y=w748) -> (x-y=→"hdt.o.ticksPerPixel":u32)
      }
      n378 = node-c288(w154) -> ()
      n379 = while {
        stop <- FALSE stop-if-true
        # "If ever timed out\nset to high and wait for clear"
        # "Transfer interaction data to host"
        n380 = xnode ("FIFO Method Node")("Timeout"=0) -> ("Element"=w722:i16, "Timed Out?"=w717:bool)  [unwired: 1 in, 1 out]
        n381 = Not(x=w717) -> (.not. x?=w716:bool)
        n382 = case shown="True" w716 {
          tunnel: w722 -> [_ w727]
          tunnel: [FALSE ("Timed Out?") w725] -> w721
          frame False {
          }
          frame True {
            n383 = xnode ("FIFO Method Node")("Element"=w727, "Timeout"=10) -> ("Timed Out?"=w725:bool)  [unwired: 1 in, 1 out]
          }
        }
        n384 = call "stateSwitch.vi"("disable"="hdt.int.s.clearDataLost", "enable"=w721) -> ("state"=→"hdt.int.s.dataLost":bool)  [unwired: 9 in]
      }
      n385 = while {
        stop <- FALSE stop-if-true
        # "Populate memory items for feedback from host"
        n386 = Unbundle By Name("aio.m.drive") -> ("write"=w665:bool, "index"=w664:u16, "data"=w663:i16)
        n387 = Unbundle By Name("ort.fit.m.weights") -> ("write"=w660:bool, "index"=w661:u16, "data"=w662:fxp<+,20,0>)
        n388 = case shown="True" w660 {
          tunnel: w661 -> [_ w681]
          tunnel: w662 -> [_ w680]
          frame False {
          }
          frame True {
            n389 = xnode ("Memory Method Node")("Address"=w681, "Data"=w680) -> ()  [unwired: 1 in, 1 out]
          }
        }
        n390 = case shown="True" w665 {
          tunnel: w664 -> [_ w683]
          tunnel: w663 -> [_ w682]
          frame False {
          }
          frame True {
            n391 = xnode ("Memory Method Node")("Address"=w683, "Data"=w682) -> ()  [unwired: 1 in, 1 out]
          }
        }
        n392 = Unbundle By Name("ort.fit.m.coefficients") -> ("write"=w658:bool, "index"=w657:u16, "fitCoefficients"=w655:T73)
        n393 = Unbundle By Name("fb.mot.m.motion") -> ("write"=w649:bool, "index"=w648:u16, "data"=w647:fxp<+,16,1>)
        n394 = case shown="True" w649 {
          tunnel: w648 -> [_ w675]
          tunnel: w647 -> [_ w674]
          frame False {
          }
          frame True {
            n395 = xnode ("Memory Method Node")("Address"=w675, "Data"=w674) -> ()  [unwired: 1 in, 1 out]
          }
        }
        n396 = case shown="True" w658 {
          tunnel: w657 -> [_ w679]
          tunnel: w655 -> [_ w678]
          frame False {
          }
          frame True {
            n397 = xnode ("Memory Method Node")("Address"=w679, "Data"=w678) -> ()  [unwired: 1 in, 1 out]
          }
        }
        n398 = disable-structure shown="CTLR_PROVIDE_SICM==1" {
          frame condition #0 (active) {
            n399 = Unbundle By Name("sicm.m.upMotion") -> ("write"=w669:bool, "index"=w668:u16, "data"=w670:fxp<+,16,1>)
            n400 = case shown="True" w669 {
              tunnel: w670 -> [_ w673]
              tunnel: w668 -> [_ w672]
              frame False {
              }
              frame True {
                n401 = xnode ("Memory Method Node")("Address"=w672, "Data"=w673) -> ()  [unwired: 1 in, 1 out]
              }
            }
          }
          frame condition #1 {
          }
        }
        n402 = Unbundle By Name("sid.m.motion") -> ("write"=w652:bool, "index"=w653:u16, "data"=w654:bool)
        n403 = case shown="True" w652 {
          tunnel: w653 -> [_ w677]
          tunnel: w654 -> [_ w676]
          frame False {
          }
          frame True {
            n404 = xnode ("Memory Method Node")("Address"=w677, "Data"=w676) -> ()  [unwired: 1 in, 1 out]
          }
        }
      }
      n405 = while {
        stop <- FALSE stop-if-true
        # "When all requested elements sent, raise interrupt"
        n406 = xnode ("FIFO Method Node")("Timeout"=0) -> ("Timed Out?"=w713:bool)  [unwired: 1 in, 2 out]
        n407 = case shown="False" w713 {
          frame False {
            n408 = call <vilib>:"niFPGA Interrupt.vi"("IRQ Number (0)"=u8 5) -> ()  [unwired: 2 in]
          }
          frame True {
          }
        }
      }
      n409 = while {
        stop <- FALSE stop-if-true
        # "Transfer background to host"
        n410 = xnode ("Register Read")() -> ("Data"=w730:bool)  [unwired: 1 in, 1 out]
        n411 = call <instrlib>:"Detect Rising Edge.vi"("signal"=w730) -> ("edge detected"=w729:bool)  [unwired: 14 in]
        n412 = case shown="True" w729 {
          frame False {
          }
          frame True {
            n413 = call <vilib>:"niFPGA Interrupt.vi"("IRQ Number (0)"=u8 4) -> ()  [unwired: 2 in]
          }
        }
      }
      n414 = while {
        stop <- FALSE stop-if-true
        # "Retract on background correct to get non-interaction background"
        n415 = disable-structure shown="FPGA_TARGET_CLASS==USB_7856R_OEM||FPGA_TARGET_CLASS==USB_7856R" {
          disable-tunnel: [w764 w765 FALSE] -> w759
          frame condition #0 {
            n416 = xnode "FPGA I/O Node"() -> ("correctBackground"=w764)  [unwired: 1 in, 1 out]
          }
          frame condition #1 (active) {
            n417 = xnode ("FIFO Method Node")("Timeout"=0) -> ("Timed Out?"=w766:bool)  [unwired: 1 in, 2 out]
            n418 = Not(x=w766) -> (.not. x?=w765:bool)
          }
          frame condition #2 {
          }
        }
        n419 = Compound Arithmetic op=AND(w759, "itc.p.allowBGC") -> (w757:bool)
        n420 = Compound Arithmetic op=OR(w757, "ort.bgc.p.start") -> (w760:bool)
        n421 = call "ort_bgc_hypervisor.vi"("ort.bgc.p.waitTicks"="ort.bgc.p.waitTicks", "ort.bgc.p.scannerTc"="ort.bgc.p.scannerTc", "start"=w760) -> ()  [unwired: 9 in]
      }
      n422 = node-c288(w164) -> ()
      n423 = disable-structure shown="FPGA_TARGET_CLASS==USB_7856R_OEM||FPGA_TARGET_CLASS==USB_7856R" {
        frame condition #0 (active) {
          n424 = disable-structure shown="FPGA_TARGET_CLASS==USB_7856R" {
            disable-tunnel: [refnum<k21> "160MHz" ("Source Name") refnum<k21> "40 MHz Onboard Clock" ("Source Name")] -> w168
            frame condition #0 {
            }
            frame condition #1 (active) {
            }
          }
          n425 = node-c288(w168) -> (w170:T44)
          n426 = timed-loop {
            timing: w170 -> [_]
            timing-out: [_] -> w169
            stop <- _ stop-if-true
            n427 = xnode ("Register Read")() -> ("Data"=w173:bool)  [unwired: 1 in, 1 out]
            n428 = call "circularCounter_v2.vi"("doStep"=TRUE, "maxCount"="aio.p.fastADCclockdec") -> ("maxPulse"=w179:bool)  [unwired: 6 in, 3 out]
            n429 = feedback #35() -> (w178:bool)  [unwired: 1 in]
            n430 = Not(x=w178) -> (.not. x?=w174:bool)
            n431 = feedback-in #35(w174, w179) -> ()
            n432 = Compound Arithmetic op=AND(w178, w179) -> (w175:bool)
            n433 = case shown="True" w173 {
              tunnel: w174 -> [_ w180]
              frame False {
              }
              frame True {
                n434 = disable-structure shown="FPGA_TARGET_CLASS==USB_7856R" {
                  disable-tunnel: w180 -> [w181 w182]
                  frame condition #0 (active) {
                    n435 = xnode "FPGA I/O Node"("Connector2/DIO0"=w181, "Connector3/DIO0"=w181) -> ()  [unwired: 2 in, 2 out]
                  }
                  frame condition #1 {
                    n436 = xnode "FPGA I/O Node"("Connector0/DIO16"=w182, "Connector0/DIO0"=w182) -> ()  [unwired: 2 in, 2 out]
                  }
                }
              }
            }
            n437 = case shown="True" w175 {
              frame False {
              }
              frame True {
                n438 = disable-structure shown="FPGA_TARGET_CLASS==USB_7856R_OEM, Default" {
                  disable-tunnel: [w236 w251] -> w184
                  disable-tunnel: [w235 w250] -> w203
                  disable-tunnel: [w234 w249] -> w202
                  disable-tunnel: [w233 w248] -> w201
                  disable-tunnel: [w232 w247] -> w200
                  disable-tunnel: [w231 w246] -> w199
                  disable-tunnel: [w230 w245] -> w198
                  disable-tunnel: [w229 w244] -> w197
                  disable-tunnel: [w228 w243] -> w196
                  disable-tunnel: [w227 w242] -> w195
                  disable-tunnel: [w226 w241] -> w194
                  disable-tunnel: [w225 w240] -> w193
                  disable-tunnel: [w224 w239] -> w192
                  disable-tunnel: [w223 w238] -> w191
                  disable-tunnel: [w222 w237] -> w186
                  frame condition #0 (active) {
                    n439 = xnode "FPGA I/O Node"() -> ("Connector2/DIO1"=w236:bool, "Connector2/DIO2"=w235:bool, "Connector2/DIO3"=w234:bool, "Connector2/DIO4"=w233:bool, "Connector2/DIO5"=w232:bool, "Connector2/DIO6"=w231:bool, "Connector2/DIO7"=w230:bool, "Connector2/DIO8"=w229:bool, "Connector2/DIO9"=w228:bool, "Connector2/DIO10"=w227:bool, "Connector2/DIO11"=w226:bool, "Connector2/DIO12"=w225:bool, "Connector2/DIO13"=w224:bool, "Connector2/DIO14"=w223:bool, "Connector2/DIO15"=w222:bool)  [unwired: 15 in, 15 out]
                  }
                  frame condition #1 {
                    n440 = xnode "FPGA I/O Node"() -> ("Connector0/DIO1"=w251, "Connector0/DIO2"=w250, "Connector0/DIO3"=w249, "Connector0/DIO4"=w248, "Connector0/DIO5"=w247, "Connector0/DIO6"=w246, "Connector0/DIO7"=w245, "Connector0/DIO8"=w244, "Connector0/DIO9"=w243, "Connector0/DIO10"=w242, "Connector0/DIO11"=w241, "Connector0/DIO12"=w240, "Connector0/DIO13"=w239, "Connector0/DIO14"=w238, "Connector0/DIO15"=w237)  [unwired: 15 in, 15 out]
                  }
                }
                n441 = xnode ("FIFO Method Node")("Timeout"=0) -> ("Element"=w221:i16)  [unwired: 1 in, 2 out]
                n442 = Number To Boolean Array(number=w221) -> (Boolean array=w219:bool[])
                n443 = Index Array(array=w219) -> (element #2=w205:bool, element #3=w206:bool, element #4=w207:bool, element #5=w208:bool, element #6=w209:bool, element #7=w210:bool, element #8=w211:bool, element #9=w212:bool, element #10=w213:bool, element #11=w214:bool, element #12=w215:bool, element #13=w216:bool, element #14=w217:bool, element #15=w218:bool, element #16=w220:bool)  [unwired: 16 in, 1 out]
                n444 = Not(x=w220) -> (.not. x?=w185:bool)
                n445 = Build Array(FALSE, w184, w203, w202, w201, w200, w199, w198, w197, w196, w195, w194, w193, w192, w191, w186) -> (w190:bool[])
                n446 = Boolean Array To Number(Boolean array=w190) -> (number=w189:u16)
                n447 = disable-structure shown="FPGA_TARGET_CLASS==USB_7856R_OEM, Default" {
                  disable-tunnel: w218 -> [w266 w281]
                  disable-tunnel: w217 -> [w265 w280]
                  disable-tunnel: w216 -> [w264 w279]
                  disable-tunnel: w215 -> [w263 w278]
                  disable-tunnel: w214 -> [w262 w277]
                  disable-tunnel: w213 -> [w261 w276]
                  disable-tunnel: w212 -> [w260 w275]
                  disable-tunnel: w211 -> [w259 w274]
                  disable-tunnel: w210 -> [w258 w273]
                  disable-tunnel: w209 -> [w257 w272]
                  disable-tunnel: w208 -> [w256 w271]
                  disable-tunnel: w207 -> [w255 w270]
                  disable-tunnel: w206 -> [w254 w269]
                  disable-tunnel: w205 -> [w253 w268]
                  disable-tunnel: w185 -> [w252 w267]
                  frame condition #0 (active) {
                    n448 = xnode "FPGA I/O Node"("Connector3/DIO15"=w253, "Connector3/DIO14"=w254, "Connector3/DIO13"=w255, "Connector3/DIO12"=w256, "Connector3/DIO11"=w257, "Connector3/DIO10"=w258, "Connector3/DIO9"=w259, "Connector3/DIO8"=w260, "Connector3/DIO7"=w261, "Connector3/DIO6"=w262, "Connector3/DIO5"=w263, "Connector3/DIO4"=w264, "Connector3/DIO3"=w265, "Connector3/DIO2"=w266, "Connector3/DIO1"=w252) -> ()  [unwired: 15 in, 15 out]
                  }
                  frame condition #1 {
                    n449 = xnode "FPGA I/O Node"("Connector0/DIO31"=w268, "Connector0/DIO30"=w269, "Connector0/DIO29"=w270, "Connector0/DIO28"=w271, "Connector0/DIO27"=w272, "Connector0/DIO26"=w273, "Connector0/DIO25"=w274, "Connector0/DIO24"=w275, "Connector0/DIO23"=w276, "Connector0/DIO22"=w277, "Connector0/DIO21"=w278, "Connector0/DIO20"=w279, "Connector0/DIO19"=w280, "Connector0/DIO18"=w281, "Connector0/DIO17"=w267) -> ()  [unwired: 15 in, 15 out]
                  }
                }
                n450 = To Word Integer(number=w189) -> (16bit integer=w188:i16)
                n451 = xnode ("FIFO Method Node")("Element"=w188, "Timeout"=0) -> ()  [unwired: 1 in, 2 out]
              }
            }
          }
          n452 = node-c288(w169) -> ()
        }
        frame condition #1 {
        }
      }
      n453 = disable-structure shown="FPGA_TARGET_CLASS==USB_7856R_OEM||FPGA_TARGET_CLASS==USB_7856R" {
        frame condition #0 {
        }
        frame condition #1 (active) {
          n454 = while {
            stop <- FALSE stop-if-true
            n455 = xnode ("FIFO Method Node")("Timeout"=0) -> ("Element"=w444:cluster{"a":i16, "b":i16})  [unwired: 1 in, 2 out]
            n456 = xnode ("Register Read")() -> ("Data"=w437:bool[])  [unwired: 1 in, 1 out]
            n457 = Unbundle(w444) -> ("a"=w436:i16, "b"=w435:i16)
            n458 = node-c288() -> (w439:T44)
            n459 = timed-loop {
              timing: w439 -> [_]
              timing-out: [_] -> w438
              tunnel: w437 -> [w457]
              tunnel: w436 -> [w453]
              tunnel: w435 -> [w452]
              tunnel: [w451] -> w434
              tunnel: [w450] -> w433
              stop <- TRUE stop-if-true
              w456 = FALSE
              n460 = Index Array(array=w457, index #1=2 ("index"), index #2=3 ("index")) -> (element #1=w455:bool, element #2=w454:bool)
              n461 = call "invert_and_blank_caseStruct.vi"("zeroOutput"=w456, "invert"=w455, "input"=w453) -> ("output"=w451:i16)  [unwired: 8 in]
              n462 = call "invert_and_blank_caseStruct.vi"("zeroOutput"=w456, "invert"=w454, "input"=w452) -> ("output"=w450:i16)  [unwired: 8 in]
            }
            n463 = node-c288(w438) -> ()
            n464 = disable-structure shown="FPGA_TARGET_CLASS==USB_7856R_OEM, Default" {
              disable-tunnel: w434 -> [w447 w449]
              disable-tunnel: w433 -> [w446 w448]
              frame condition #0 {
                n465 = xnode "FPGA I/O Node"("Connector1/AO2"=w447, "Connector1/AO3"=w446) -> ()  [unwired: 2 in, 2 out]
              }
              frame condition #1 (active) {
                n466 = xnode "FPGA I/O Node"("Connector0/AO2"=w449, "Connector0/AO3"=w448) -> ()  [unwired: 2 in, 2 out]
              }
            }
            n467 = call "Tick Count5"() -> ("Tick Count(Ticks)"=w441:u32)
            n468 = feedback #36() -> (w442:u32)  [unwired: 1 in]
            n469 = feedback-in #36(w441) -> ()
            n470 = Subtract(x=w441, y=w442) -> (x-y=→"aio.s.slowActualFBOutRate":u32)
          }
        }
        frame condition #2 {
        }
      }
      n471 = while {
        stop <- FALSE stop-if-true
        # "z Watchdog for auto-approach"
        n472 = xnode ("Register Read")() -> ("Data"=w302:bool)  [unwired: 1 in, 1 out]
        n473 = call <instrlib>:"Detect Rising Edge.vi"("signal"=w302) -> ("edge detected"=w301:bool)  [unwired: 14 in]
        n474 = Compound Arithmetic op=AND(w301, "fb.zWatchdogArm") -> (w303:bool)
        n475 = case shown="True" w303 {
          frame False {
          }
          frame True {
            n476 = local write "fb.zWatchdogArm"(FALSE ("fb.zWatchdogArm")) -> ()
            n477 = call <vilib>:"niFPGA Interrupt.vi"("IRQ Number (0)"=u8 8) -> ()  [unwired: 2 in]
          }
        }
      }
      n478 = node-c288(w166) -> ()
      n479 = while {
        stop <- FALSE stop-if-true
        # "Local wave recording hypervisor for ORT"
        n480 = call "lwr_hypervisor.vi"("lwr.p.start"="lwr.p.start") -> ()  [unwired: 11 in]
      }
      n481 = node-c288(w158) -> ()
    }
    frame condition #1 {
    }
  }
  n482 = disable-structure shown="CTLR_PROVIDE_SCAN==1" {
    frame condition #0 (active) {
      n483 = node-c288() -> (w781:T44)  [unwired: 1 in]
      n484 = timed-loop {
        timing: w781 -> [_]
        timing-out: [_] -> w780
        stop <- _ stop-if-true
        n485 = call "dio_pixelSync.vi"() -> ()  [unwired: 12 in]
      }
      n486 = node-c288(w780) -> ()
      n487 = node-c288(refnum<k21> "5MHz" ("Source Name")) -> (w784:T44)
      n488 = timed-loop {
        timing: w784 -> [_]
        timing-out: [_] -> w783
        stop <- _ stop-if-true
        w790 = TRUE ("Ready for Output")
        # "0- never\n1- end of line\n2- end of frame"
        # "Automatic background correct request"
        n489 = xnode ("FIFO Method Node")("Ready for Output"=w790) -> ("Output Valid"=w791:bool)  [unwired: 1 in, 2 out]
        n490 = xnode ("FIFO Method Node")("Ready for Output"=w790) -> ("Output Valid"=w789:bool)  [unwired: 1 in, 2 out]
        n491 = case shown="2" "ort.bgc.requestType" {
          tunnel: [FALSE w798 w799] -> w792
          tunnel: w789 -> [_ w798 _]
          tunnel: w791 -> [_ _ w799]
          frame 0, Default {
          }
          frame 1 {
          }
          frame 2 {
          }
        }
        n492 = disable-structure shown="Default" {
          disable-tunnel: w792 -> [w794 w795 _]
          frame condition #0 {
            n493 = xnode "FPGA I/O Node"("correctBackground"=w794) -> ()  [unwired: 1 in, 1 out]
          }
          frame condition #1 (active) {
            n494 = xnode ("FIFO Method Node")("Element"=TRUE, "Input Valid"=w795) -> ()  [unwired: 1 in, 2 out]
          }
          frame condition #2 {
          }
        }
      }
      n495 = node-c288(w783) -> ()
      n496 = while {
        stop <- FALSE stop-if-true
        # "x-y physical output"
        n497 = call "Tick Count3"() -> ("Tick Count(Ticks)"=w815:u32)
        n498 = xnode ("FIFO Method Node")("Timeout"=-1) -> ("Element"=w817:cluster{"x":i16, "y":i16})  [unwired: 1 in, 2 out]
        n499 = feedback-in #37(w815) -> ()
        n500 = feedback #37() -> (w814:u32)  [unwired: 1 in]
        n501 = Subtract(x=w815, y=w814) -> (x-y=→"se.s.realXYOutputRate":u32)
        n502 = Unbundle By Name(w817) -> ("x"=w810:i16, "y"=w809:i16)
        n503 = xnode ("Register Read")() -> ("Data"=w806:bool[])  [unwired: 1 in, 1 out]
        n504 = node-c288() -> (w812:T44)
        n505 = timed-loop {
          timing: w812 -> [_]
          timing-out: [_] -> w811
          tunnel: w810 -> [w828]
          tunnel: w809 -> [w827]
          tunnel: [w826] -> w808
          tunnel: [w825] -> w807
          tunnel: w806 -> [w832]
          stop <- TRUE stop-if-true
          w829 = FALSE
          n506 = Index Array(array=w832, index #1=0 ("index"), index #2=1 ("index")) -> (element #1=w824:bool, element #2=w823:bool)
          n507 = call "invert_and_blank_caseStruct.vi"("zeroOutput"=w829, "invert"=w824, "input"=w828) -> ("output"=w826:i16)  [unwired: 8 in]
          n508 = call "invert_and_blank_caseStruct.vi"("zeroOutput"=w829, "invert"=w823, "input"=w827) -> ("output"=w825:i16)  [unwired: 8 in]
        }
        n509 = node-c288(w811) -> ()
        n510 = disable-structure shown="FPGA_TARGET_CLASS==USB_7856R_OEM||FPGA_TARGET_CLASS==USB_7851R||FPGA_TARGET_CLASS==USB_7841R, Default" {
          disable-tunnel: w808 -> [w820 w822]
          disable-tunnel: w807 -> [w819 w821]
          frame condition #0 {
            n511 = xnode "FPGA I/O Node"("Connector1/AO0"=w820) -> ()  [unwired: 1 in, 1 out]
            n512 = xnode "FPGA I/O Node"("Connector1/AO1"=w819) -> ()  [unwired: 1 in, 1 out]
          }
          frame condition #1 (active) {
            n513 = xnode "FPGA I/O Node"("Connector0/AO0"=w822) -> ()  [unwired: 1 in, 1 out]
            n514 = xnode "FPGA I/O Node"("Connector0/AO1"=w821) -> ()  [unwired: 1 in, 1 out]
          }
        }
      }
    }
    frame condition #1 {
    }
  }
  n515 = disable-structure shown="CTLR_PROVIDE_SCAN==1" {
    frame condition #0 (active) {
      n516 = node-c288() -> (w839:T44)  [unwired: 1 in]
      n517 = disable-structure shown="FPGA_TARGET_CLASS==USB_7856R_OEM||FPGA_TARGET_CLASS==USB_7856R" {
        frame condition #0 (active) {
          n518 = while {
            stop <- FALSE stop-if-true
            w860 = 0 ("Timeout")
            # "Triggers End of Line / Frame"
            n519 = xnode ("FIFO Method Node")("Timeout"=w860) -> ("Timed Out?"=w866:bool)  [unwired: 1 in, 2 out]
            n520 = xnode ("FIFO Method Node")("Timeout"=w860) -> ("Timed Out?"=w864:bool)  [unwired: 1 in, 2 out]
            n521 = xnode ("FIFO Method Node")("Timeout"=w860) -> ("Timed Out?"=w862:bool)  [unwired: 1 in, 2 out]
            n522 = Not(x=w864) -> (.not. x?=w863:bool)
            n523 = Not(x=w866) -> (.not. x?=w865:bool)
            n524 = Not(x=w862) -> (.not. x?=w861:bool)
            n525 = xnode "FPGA I/O Node"("BeginningOfFrame"=w861, "EndOfLine"=w863, "EndOfFrame"=w865) -> ()  [unwired: 3 in, 3 out]
          }
          n526 = node-c288() -> (w843:T44)  [unwired: 1 in]
          n527 = timed-loop {
            timing: w843 -> [_]
            timing-out: [_] -> w842
            stop <- _ stop-if-true
            # "Need to initialize initialPosition somewhere"
            # "Only one axis is modified at a time, the remaining two are copied from the previous value"
            # "Write a Sawtooth Waveform to 3 FIFOs (Stick-Slip)"
            n528 = call "waveformGerneratorStickSlip_v3.vi"("Ramp range"="wfm.rampRange", "Parameters"="wfm.Parameters", "InitialPositions"="wfm.initialPositions", "Reset"="wfm.reset") -> ("DisplacementFinished"=→"wfm.displacementFinished":bool, "MicroStepIndex"=→"wfm.microStepIndex":cluster{"CurrentUstep":i16, "NextUstep":i16}, "RampIndex"=→"wfm.rampIndex":cluster{"ramp index":i16, "NextRamp":i16}, "Outputs"=w848:T74)  [unwired: 8 in]
            n529 = Unbundle By Name(w848) -> ("Xout"=w847:fxp<+/-,16,16>, "Yout"=w845:fxp<+/-,16,16>, "Zout"=w846:fxp<+/-,16,16>, "OutputValid"=w844:bool)
            n530 = xnode ("FIFO Write Using Handshaking")("Element"=w847, "Input Valid"=w844) -> ()  [unwired: 1 in, 2 out]
            n531 = xnode ("FIFO Write Using Handshaking")("Element"=w845, "Input Valid"=w844) -> ()  [unwired: 1 in, 2 out]
            n532 = xnode ("FIFO Write Using Handshaking")("Element"=w846, "Input Valid"=w844) -> ()  [unwired: 1 in, 2 out]
          }
          n533 = node-c288(w842) -> ()
          n534 = while {
            stop <- FALSE stop-if-true
            w877 = 0
            # "Generate variable voltages"
            # "Slow host-controlled signal generator"
            n535 = Index Array(array="aio.o.outputs") -> (element #1=w882:i16, element #2=w874:i16, element #3=w872:i16, element #4=w870:i16)  [unwired: 4 in]
            n536 = xnode ("FIFO Read")("Timeout"=w877) -> ("Element"=w880:fxp<+/-,16,16>)  [unwired: 1 in, 2 out]
            n537 = xnode ("FIFO Read")("Timeout"=w877) -> ("Element"=w879:fxp<+/-,16,16>)  [unwired: 1 in, 2 out]
            n538 = xnode ("FIFO Read")("Timeout"=w877) -> ("Element"=w878:fxp<+/-,16,16>)  [unwired: 1 in, 2 out]
            n539 = call "Tick Count2"() -> ("Tick Count(Ticks)"=w876:u32)
            n540 = feedback #38() -> (w875:u32)  [unwired: 1 in]
            n541 = feedback-in #38(w876) -> ()
            n542 = Select(t=w880, s="aio.wfm.enable", f=w874) -> (s? t:f=w873:fxp<+/-,16,16>)
            n543 = Select(t=w879, s="aio.wfm.enable", f=w872) -> (s? t:f=w871:fxp<+/-,16,16>)
            n544 = Select(t=w878, s="aio.wfm.enable", f=w870) -> (s? t:f=w869:fxp<+/-,16,16>)
            n545 = Subtract(x=w876, y=w875) -> (x-y=→"aio.s.slowActualOutputRate":u32)
            n546 = disable-structure shown="FPGA_TARGET_CLASS==USB_7856R_OEM||FPGA_TARGET_CLASS==PXI_7841R||FPGA_TARGET_CLASS==PXI_7856R, Default" {
              disable-tunnel: w882 -> [w888 w892]
              disable-tunnel: w873 -> [w887 w891]
              disable-tunnel: w871 -> [w886 w890]
              disable-tunnel: w869 -> [w885 w889]
              frame condition #0 {
                n547 = xnode "FPGA I/O Node"("Connector1/AO4"=w888, "Connector1/AO5"=w887, "Connector1/AO6"=w886, "Connector1/AO7"=w885) -> ()  [unwired: 4 in, 4 out]
              }
              frame condition #1 (active) {
                n548 = xnode "FPGA I/O Node"("Connector0/AO4"=w892, "Connector0/AO5"=w891, "Connector0/AO6"=w890, "Connector0/AO7"=w889) -> ()  [unwired: 4 in, 4 out]
              }
            }
          }
        }
        frame condition #1 {
        }
      }
      n549 = timed-loop {
        timing: w839 -> [_]
        timing-out: [_] -> w838
        stop <- _ stop-if-true
        n550 = xnode ("FIFO Method Node")("Timeout"=0) -> ("Element"=w909:i16[], "Timed Out?"=w897:bool)  [unwired: 1 in, 1 out]
        n551 = Index Array(array=w909) -> (element #1=w920:i16, element #2=w919:i16, element #3=w918:i16, element #4=w917:i16, element #5=w916:i16, element #6=w915:i16, element #7=w914:i16, element #8=w913:i16)  [unwired: 8 in]
        n552 = Not(x=w897) -> (.not. x?=w896:bool)
        n553 = disable-structure shown="FPGA_TARGET_CLASS==USB_7856R_OEM||FPGA_TARGET_CLASS==USB_7856R" {
          disable-tunnel: w920 -> [w926 _]
          disable-tunnel: w919 -> [w925 _]
          disable-tunnel: w896 -> [w923 _]
          frame condition #0 (active) {
            n554 = Bundle("Numeric"=w926, "Numeric"=w925) -> (w924:cluster{"Numeric":i16, "Numeric":i16})  [unwired: 1 in]
            n555 = xnode ("FIFO Method Node")("Element"=w924, "Input Valid"=w923) -> ()  [unwired: 1 in, 2 out]
          }
          frame condition #1 {
          }
        }
        n556 = xnode ("Register Read")() -> ("Data"=w908:bool[])  [unwired: 1 in, 1 out]
        n557 = Index Array(array=w908) -> (element #1=w907:bool, element #2=w906:bool, element #3=w905:bool, element #4=w904:bool, element #5=w903:bool, element #6=w902:bool, element #7=w901:bool)  [unwired: 7 in]
        n558 = call "invert_and_blank_caseStruct.vi"("invert"=w907, "input"=w920) -> ("output"=→"aio.s.slowVertical":i16)  [unwired: 9 in]
        n559 = call "invert_and_blank_caseStruct.vi"("invert"=w906, "input"=w919) -> ("output"=→"aio.s.slowHoriz":i16)  [unwired: 9 in]
        n560 = call "invert_and_blank_caseStruct.vi"("invert"=w905, "input"=w918) -> ("output"=→"aio.s.sum":i16)  [unwired: 9 in]
        n561 = call "invert_and_blank_caseStruct.vi"("invert"=w904, "input"=w917) -> ("output"=w894:i16)  [unwired: 9 in]
        n562 = call "invert_and_blank_caseStruct.vi"("invert"=w903, "input"=w916) -> ("output"=w895:i16)  [unwired: 9 in]
        n563 = call "invert_and_blank_caseStruct.vi"("invert"=w902, "input"=w915) -> ("output"=w900:i16)  [unwired: 9 in]
        n564 = call "invert_and_blank_caseStruct.vi"("input"=w914) -> ("output"=w899:i16)  [unwired: 10 in]
        n565 = call "invert_and_blank_caseStruct.vi"("invert"=w901, "input"=w913) -> ("output"=w898:i16)  [unwired: 9 in]
        n566 = Build Array(w894, w895, w900, w899, w898) -> (w922:i16[])
        "aio.o.inputs" <- w922
        n567 = Bundle("output"=w894, "output"=w895) -> (w893:cluster{"output":i16, "output":i16})  [unwired: 1 in]
        n568 = xnode ("FIFO Write")("Element"=w893, "Input Valid"=w896) -> ()  [unwired: 1 in, 2 out]
        n569 = xnode ("FIFO Method Node")("Element"=w922, "Input Valid"=w896) -> ()  [unwired: 1 in, 2 out]
      }
      n570 = while {
        stop <- FALSE stop-if-true
        w983 = i16 0
        # "Pad with zeroes until we find a \nbetter use for these 3 channels"
        # "input recording and passover to averaging"
        n571 = xnode ("FIFO Method Node")("Timeout"=-1) -> ("Element"=w982:i16[])  [unwired: 1 in, 2 out]
        n572 = Build Array(w983, w983, w983) -> (w981:i16[])
        n573 = Build Array (concatenate)(w982, w981) -> (w980:i16[])
        n574 = xnode "Reinterpret Number"("x"=w980) -> ("y"=w985:fxp<+/-,16,1>[])
        n575 = xnode ("FIFO Method Node")("Element"=w985, "Timeout"=0) -> ()  [unwired: 1 in, 2 out]
      }
      n576 = while {
        stop <- FALSE stop-if-true
        # "Output to host"
        n577 = xnode ("FIFO Method Node")("Timeout"=-1) -> ("Element"=w975:fxp<+/-,22,1>[])  [unwired: 1 in, 2 out]
        n578 = for {
          tunnel: w975 -> [w979] mode=indexing
          n579 = xnode ("FIFO Method Node")("Element"=w979, "Timeout"=0) -> ()  [unwired: 1 in, 2 out]
        }
      }
      n580 = node-c288(w838) -> ()
      n581 = node-c288() -> (w841:T44)  [unwired: 1 in]
      n582 = timed-loop {
        timing: w841 -> [_]
        timing-out: [_] -> w840
        stop <- _ stop-if-true
        # "Output averaging and pixel synchronous output"
        n583 = disable-structure shown="FPGA_TARGET_CLASS==STORAGE" {
          disable-tunnel: "hdt.aux.o.enable" -> [w963 w965]
          frame condition #0 (active) {
            n584 = call "hdt_aux_averageChannels.vi"("enableOutput"=w963) -> ()  [unwired: 11 in]
          }
          frame condition #1 {
            w970 = TRUE ("Ready for Output")
            n585 = xnode ("FIFO Method Node")("Ready for Output"=w970) -> ("Output Valid"=w966:bool)  [unwired: 1 in, 2 out]
            n586 = xnode ("FIFO Method Node")("Ready for Output"=w970) -> ("Element"=w969:fxp<+/-,22,1>[], "Output Valid"=w968:bool)  [unwired: 1 in, 1 out]
            n587 = feedback-in #39(w969, w968) -> ()
            n588 = feedback #39() -> (w967:fxp<+/-,22,1>[])  [unwired: 1 in]
            n589 = Compound Arithmetic op=AND(w966, w965) -> (w964:bool)
            n590 = xnode ("FIFO Method Node")("Element"=w967, "Input Valid"=w964) -> ()  [unwired: 1 in, 2 out]
          }
        }
      }
      n591 = while {
        stop <- FALSE stop-if-true
        n592 = disable-structure shown="FPGA_TARGET_CLASS==USB_7856R_OEM||FPGA_TARGET_CLASS==PXI_7841R||FPGA_TARGET_CLASS==USB_7851R" {
          disable-tunnel: [w953 w961 _] -> w934
          disable-tunnel: [w952 w960 _] -> w935
          disable-tunnel: [w951 w959 _] -> w936
          disable-tunnel: [w950 w958 _] -> w937
          disable-tunnel: [w949 w957 _] -> w938
          disable-tunnel: [w948 w956 _] -> w933
          disable-tunnel: [w947 w955 _] -> w940
          disable-tunnel: [w946 w954 _] -> w939
          frame condition #0 {
            n593 = xnode "FPGA I/O Node"() -> ("Connector1/AI0"=w947, "Connector1/AI1"=w946, "Connector1/AI2"=w949, "Connector1/AI3"=w950, "Connector1/AI4"=w951, "Connector1/AI5"=w952, "Connector1/AI6"=w953, "Connector1/AI7"=w948)  [unwired: 8 in, 8 out]
          }
          frame condition #1 (active) {
            n594 = xnode "FPGA I/O Node"() -> ("Connector0/AI0"=w955:i16, "Connector0/AI1"=w954:i16, "Connector0/AI2"=w957:i16, "Connector0/AI3"=w958:i16, "Connector0/AI4"=w959:i16, "Connector0/AI5"=w960:i16, "Connector0/AI6"=w961:i16, "Connector0/AI7"=w956:i16)  [unwired: 8 in, 8 out]
          }
          frame condition #2 {
          }
        }
        n595 = call "Tick Count4"() -> ("Tick Count(Ticks)"=w941:u32)
        n596 = feedback #40() -> (w942:u32)  [unwired: 1 in]
        n597 = feedback-in #40(w941) -> ()
        n598 = Subtract(x=w941, y=w942) -> (x-y=→"aio.s.slowActualInputRate":u32)
        n599 = Build Array(w940, w939, w938, w937, w936, w935, w934, w933) -> (w932:i16[])
        n600 = xnode ("FIFO Method Node")("Element"=w932, "Timeout"=0) -> ()  [unwired: 1 in, 2 out]
        n601 = call "Loop Timer"("Count(Ticks)"="aio.i.slowInputRate") -> ()  [unwired: 1 out]
      }
      n602 = node-c288(w840) -> ()
    }
    frame condition #1 {
    }
  }
  n603 = disable-structure shown="FPGA_TARGET_CLASS==PXI_7851R||FPGA_TARGET_CLASS==PXI_7841R||FPGA_TARGET_CLASS==USB_7856R_OEM||FPGA_TARGET_CLASS==USB_7856R" {
    frame condition #0 (active) {
      n604 = while {
        stop <- FALSE stop-if-true
        # "Output the Step Motor state"
        n605 = xnode ("Memory Method Node")("Address"="smd.address") -> ("Data"=w995:bool[])  [unwired: 1 in, 1 out]
        n606 = Not(x=w995) -> (.not. x?=w994:bool[])
        n607 = Array To Cluster(array=w994) -> (cluster=w993:T75)
        n608 = Unbundle By Name(w993) -> ("[0]"=w992:bool, "[1]"=w991:bool, "[2]"=w990:bool, "[3]"=w989:bool)
        n609 = disable-structure shown="FPGA_TARGET_CLASS==PXI_7851R||FPGA_TARGET_CLASS==PXI_7841R" {
          disable-tunnel: w992 -> [w1000 w1004]
          disable-tunnel: w991 -> [w999 w1003]
          disable-tunnel: w990 -> [w998 w1002]
          disable-tunnel: w989 -> [w997 w1001]
          frame condition #0 (active) {
            n610 = xnode "FPGA I/O Node"("A"=w1000, "B"=w999, "C"=w998, "D"=w997) -> ()  [unwired: 4 in, 4 out]
          }
          frame condition #1 {
            n611 = xnode "FPGA I/O Node"("Connector0/DIO0"=w1004, "Connector0/DIO1"=w1003, "Connector0/DIO2"=w1002, "Connector0/DIO3"=w1001) -> ()  [unwired: 4 in, 4 out]
          }
        }
      }
    }
    frame condition #1 {
    }
  }
  n612 = disable-structure shown="FPGA_TARGET_CLASS==USB_7856R_OEM||FPGA_TARGET_CLASS==USB_7856R" {
    frame condition #0 (active) {
      n613 = while {
        stop <- FALSE stop-if-true
        # "Stepper Motor Driver Interface (Enable, Direction and Step)"
        n614 = feedback #41() -> (w1015:bool)  [unwired: 1 in]
        n615 = call "circularCounter_v2.vi"("reset"="stepmot.on", "doStep"=w1015, "maxCount"="stepmot.steps") -> ("maxReached"=w1016:bool)  [unwired: 5 in, 3 out]
        n616 = Not(x=w1016) -> (.not. x?=w1014:bool)
        "stepmot.running" <- w1014
        n617 = feedback-in #41(w1014) -> ()
        n618 = case shown="True" w1014 {
          frame False {
          }
          frame True {
            n619 = flat-sequence {
              tunnel: "stepmot.delay(ms)" -> [w1022]
              tunnel: "stepmot.delay(ms)" -> [w1024]
              frame #0 {
                n620 = xnode "FPGA I/O Node"("stepmot.steps"=TRUE) -> ()  [unwired: 1 in, 1 out]
              }
              frame #1 {
                n621 = call "Wait"("Count(mSec)"=w1022) -> ()  [unwired: 1 out]
              }
              frame #2 {
                n622 = xnode "FPGA I/O Node"("stepmot.steps"=FALSE) -> ()  [unwired: 1 in, 1 out]
              }
              frame #3 {
                n623 = call "Wait2"("Count(mSec)"=w1024) -> ()  [unwired: 1 out]
              }
            }
          }
        }
        n624 = case shown="True" "stepmot.on" {
          frame False {
          }
          frame True {
            n625 = local write "stepmot.on"(FALSE ("stepmot.on")) -> ()
          }
        }
      }
      n626 = node-c288() -> (w1006:T44)  [unwired: 1 in]
      n627 = timed-loop {
        timing: w1006 -> [_]
        timing-out: [_] -> w1005
        stop <- _ stop-if-true
        n628 = xnode "FPGA I/O Node"("stepmot.enable"="stepmot.enable", "stepmot.direction"="stepmot.dir") -> ()  [unwired: 2 in, 2 out]
      }
      n629 = node-c288(w1005) -> ()
    }
    frame condition #1 {
    }
  }
  n630 = disable-structure shown="FPGA_TARGET_CLASS==USB_7856R||FPGA_TARGET_CLASS==USB_7856R_OEM||FPGA_TARGET_CLASS==PXI_7851R" {
    frame condition #0 (active) {
      # "Sync Reset Data Out"
      n631 = while {
        stop <- FALSE stop-if-true
        # "Multplexer"
        n632 = xnode ("Register Write")("Data"="dio.p.multiplexerOE") -> ()  [unwired: 1 in, 1 out]
        n633 = xnode ("Register Write")("Data"="dio.i.dataIn") -> ()  [unwired: 1 in, 1 out]
        n634 = xnode ("Register Write")("Data"="dio.p.multiplexerclock") -> ()  [unwired: 1 in, 1 out]
      }
      n635 = node-c288() -> (w1026:T44)  [unwired: 1 in]
      n636 = timed-loop {
        timing: w1026 -> [_]
        timing-out: [_] -> w1025
        stop <- _ stop-if-true
        n637 = xnode ("Register Read")() -> ("Data"=w1034:bool)  [unwired: 1 in, 1 out]
        n638 = xnode ("Register Read")() -> ("Data"=w1035:bool)  [unwired: 1 in, 1 out]
        n639 = xnode ("Register Read")() -> ("Data"=w1031:bool)  [unwired: 1 in, 1 out]
        n640 = disable-structure shown="FPGA_TARGET_CLASS==USB_7856R_OEM, Default" {
          disable-tunnel: w1035 -> [w1040 _]
          disable-tunnel: w1034 -> [w1039 _]
          disable-tunnel: "dio.p.multiplexerSync" -> [w1038 _]
          disable-tunnel: "dio.p.multiplexerReset" -> [w1037 _]
          disable-tunnel: w1031 -> [w1036 _]
          frame condition #0 (active) {
            n641 = xnode "FPGA I/O Node"("multiplexer.reset"=w1037, "multiplexer.oe"=w1036, "multiplexer.data"=w1039, "multiplexer.clk"=w1040, "multiplexer.sync"=w1038) -> ()  [unwired: 5 in, 5 out]
          }
          frame condition #1 {
          }
        }
      }
      n642 = node-c288(w1025) -> ()
    }
    frame condition #1 {
    }
  }
